vi "WS1050 16 DUT Reliability HD_Cycling Ver1.8.vi"() -> ()   [LabVIEW 2012]
uses:
  Type Defs/WSVCAP SHL I2C DUT Mask Mode Enum.ctl
  <vilib>/Utility/file.llb/Read From Spreadsheet File (DBL).vi
  SubVI/Agilent E363X Series/Agilent E363X Series.lvlib
  SubVI/keithley_2000/Keithley 2000/Keithley 2000.lvlib
  SubVI/2012_Keithley 24XX/Keithley 24XX.lvlib
panel:
  out "VISA resource name out":refnum<visa-resource-name>="GPIB0::3::INSTR"
  out "error out 2":errorcluster={"status"=TRUE, "code"=-63192, "source"="niLvFpga_Open_PXI-7813R.vi"}
  in  "Reg1_Bit Cntrl":string[](array[string])=["01", "02", "04", "08", "10", "20", "40", "80", "03", "06", "0C", "D8", "33", "66", "CC", "07", "0E", "1C", "38", "70", "E0", "0F", "1E", "3C", "78", "F0", "1F", "3E", "7C", "F8", "3F", "7E", "FC", "7F", "FE", "FD", "FB", "F7", "EF", "DF", "BF", "7F", "FC", "F9", "F3", "E7", "CF", "9F", "3F", "F8", "F1", "E3", "C7", "8F", "1F", "F0", "E1", "C3", "87", "0F", "E0", "C1", "83", "07", "C0", "81", "03", "AA", "55", "00"]
  out "date string":string="5/19/2014"
  out "PS1 Out":refnum<visa-resource-name>
  out "Ke2000 Out":refnum<visa-resource-name>="GPIB0::9::INSTR"
  in  "Tab Control":T1(tab)
  in  "No of Cmd":i64=3
  in  "Serial Number":string[][](table)=[["DUT", "SN"], ["DUT1", "1"], ["DUT2", "2"], ["DUT3", "3"], ["DUT4", "4"], ["DUT5", "5"], ["DUT6", "6"], ["DUT7", "7"], ["DUT8", "8"], ["DUT9", "9"], ["DUT10", "10"], ["DUT11", "11"], ["DUT12", "12"], ["DUT13", "13"], ["DUT14", "14"], ["DUT15", "15"], ["DUT16", "16"]]
  out "AD7747 Values":string[][](table)
  in  "SPI Clock Rate (Hz)":dbl=5000000.0 caption="Cycle Speed" format="%.1p Hz"
  in  "Lot#":string="3T9BB"
  in  "Wafer#":string="25-EB"
  in  "File Name":string="CYC_3T9BB_25_EB_65C_40V_50DC_BRD3_141107_1"
  in  "TMN DC\\CAP Data Log File Path":path=path "C:/WS1050 16 DUT Data"
  in  "Test Program":string="WS1050 16 DUT Reliability HD_Cycling Ver1.8"
  out "Current Date":string="8/28/2014"
  out "Current Time":string="0950"
  in  "Start Date":string="4/24/2014"
  in  "Start Time":string="1542"
  in  "Comment":string="CYC65C40V"
  in  "OK Button":bool
  in  "Calibration":bool
  in  "Verify CP":bool
  in  "CP Setting":i32(ring) items=["CP OFF", "CP ON", "CP 35V", "CP 40V", "DVA ON", "DVA OFF", "REG1 ON", "REG1 OFF", "REG2 ON", "REG2 OFF", "REG3 ON", "REG3 OFF"]
  in  "Set VDD":dbl=3.7 format="%.3g"
  in  "Command":string[](array[string])=["0702013B3B3B", "0702013B3B3B", "070201000000"]
  in  "SPI Clock Rate (Hz)":dbl=1000000.0 caption="Meas Speed" format="%.1p Hz"
  out "AR  Meas(Hz)":dbl
  in  "PS1 Source":refnum<visa-resource-name>="GPIB0::5::INSTR"
  in  "Ke2000":refnum<visa-resource-name>="GPIB0::9::INSTR"
  in  "CP to HD/Cycle":i32(ring)=1 items=["CP HDC 35V", "CP HDC 40.25V", "CP HDC 27.5V", "CP HDC 30.5V", "CP HDC 44V"]
  out "Simulate FPGA":bool
  out "Online":bool
  out "AR Cycling(Hz)":dbl=5000000.0
  in  "Ke2400":refnum<visa-resource-name>="GPIB0::3::INSTR"
  in  "Initialize AD7747":bool
  in  "DUT Mask Mode":T2=enum."All"
  in  "RFFE Slave Address":u8=7 caption="Slave Address" format="0x%02x"
  out "Activity Log":string="05/19/2014 -- 12:24:35.853::WSVCAP::APP::Application Started\n05/19/2014 -- 12:24:37.606::WSVCAP::WSVCAP SHL::WR I2C-REG:0x0A;MASK:0xFFFFFFFFFFFF;C1 DATA:22:22:22:22:22:22:22:22:22:22:22:22:22:22:22:22;C2 DATA:22:22:22:22:22:22:22:22:22:22:22:22:22:22:22:22;C3 DATA:22:22:22:22:22:22:22:22:22:22:22:22:22:22:22:22\r\n05/19/2014 -- 12:24:37.773::WSVCAP::WSVCAP SHL::WR I2C-ST:0,0,4,1\r\n05/19/2014 -- 12:24:37.903::WSVCAP::WSVCAP SHL::RD I2C-BYTES:4;ADD:0x00;MASK:0xFFFFFFFFFFFF\r\n05/19/2014 -- 12:24:38.045::WSVCAP::WSVCAP SHL::RD I2C:C1 DATA:2:2:2:2:2:2:2:2:2:2:2:2:2:2:2:2|A7:A9:AA:82:82:7F:82:81:82:81:83:82:81:82:82:81|46:36:BB:88:44:A3:E9:2B:32:20:ED:25:BB:3D:68:B|2C:6A:EB:A7:22:56:FE:CC:36:82:D7:B0:3B:48:F9:CC;C2 DATA:2:2:2:2:2:2:2:2:2:2:2:2:2:2:2:2|94:94:94:80:80:80:80:80:81:7E:7E:81:80:7E:80:80|47:33:15:82:62:B:E8:1C:D7:C3:7D:41:7C:B7:4C:2A|C4:B4:AE:8:1E:D1:4E:37:11:C0:6F:63:42:9D:63:B5;C3 DATA:2:2:2:2:2:2:2:2:2:2:2:2:2:2:2:2|95:95:95:81:81:7E:81:80:84:7D:80:83:81:7E:7F:80|AB:C4:14:B5:7B:52:DF:C9:79:5D:5F:30:99:31:1E:F4|6E:5C:F7:A8:C3:EB:7B:EF:33:92:89:77:4D:67:75:DD;STATUS:0:0:4:0\r\n05/19/2014 -- 12:24:38.046::WSVCAP::WSVCAP SHL::WR I2C-REG:0x0A;MASK:0xFFFFFFFFFFFF;C1 DATA:22:22:22:22:22:22:22:22:22:22:22:22:22:22:22:22;C2 DATA:22:22:22:22:22:22:22:22:22:22:22:22:22:22:22:22;C3 DATA:22:22:22:22:22:22:22:22:22:22:22:22:22:22:22:22\r\n05/19/2014 -- 12:24:38.089::WSVCAP::WSVCAP SHL::WR I2C-ST:0,0,4,1\r\n05/19/2014 -- 12:24:38.219::WSVCAP::WSVCAP SHL::RD I2C-BYTES:4;ADD:0x00;MASK:0xFFFFFFFFFFFF\r\n05/19/2014 -- 12:24:38.362::WSVCAP::WSVCAP SHL::RD I2C:C1 DATA:2:2:2:2:2:2:2:2:2:2:2:2:2:2:2:2|A7:AB:AA:82:82:82:83:83:82:82:82:82:7F:82:82:81|4B:32:96:83:3E:61:43:17:25:62:AB:4D:A2:40:2E:5|3C:76:2B:B4:EE:E4:A9:1A:AA:A:26:C7:21:2E:87:5B;C2 DATA:2:2:2:2:2:2:2:2:2:2:2:2:2:2:2:2|94:94:94:80:80:80:80:80:80:7F:80:81:80:80:7F:80|4A:32:19:7D:19:6C:79:46:61:7F:4B:B8:A5:30:F3:14|B4:70:A:8C:9C:DC:43:FA:1E:A:C6:21:A:A9:13:F3;C3 DATA:2:2:2:2:2:2:2:2:2:2:2:2:2:2:2:2|95:97:94:81:80:81:82:81:80:7E:81:84:7F:81:80:80|B2:32:D0:A7:9E:4C:AB:D4:EE:D9:F0:82:B7:91:7:FF|C1:91:B6:3D:D8:E:1B:4F:9F:6A:F1:6C:E7:3F:7:BA;STATUS:0:0:4:0\r\n05/19/2014 -- 12:24:38.364::WSVCAP::WSVCAP SHL::WR I2C-REG:0x0A;MASK:0xFFFFFFFFFFFF;C1 DATA:22:22:22:22:22:22:22:22:22:22:22:22:22:22:22:22;C2 DATA:22:22:22:22:22:22:22:22:22:22:22:22:22:22:22:22;C3 DATA:22:22:22:22:22:22:22:22:22:22:22:22:22:22:22:22\r\n05/19/2014 -- 12:24:38.406::WSVCAP::WSVCAP SHL::WR I2C-ST:0,0,4,1\r\n05/19/2014 -- 12:24:38.536::WSVCAP::WSVCAP SHL::RD I2C-BYTES:4;ADD:0x00;MASK:0xFFFFFFFFFFFF\r\n05/19/2014 -- 12:24:38.678::WSVCAP::WSVCAP SHL::RD I2C:C1 DATA:2:2:2:2:2:2:2:2:2:2:2:2:2:2:2:2|A7:A9:AB:82:82:81:82:82:82:82:82:82:82:82:82:81|46:71:4C:87:43:3D:7F:FC:25:4F:8E:54:97:3E:60:8C|AA:F4:1F:B5:CE:43:1F:36:9:87:9C:78:86:5:B6:8E;C2 DATA:2:2:2:2:2:2:2:2:2:2:2:2:2:2:2:2|94:94:94:80:7F:7F:80:80:80:80:80:81:80:80:80:80|49:36:18:7D:6E:C5:E4:3C:81:2E:41:D3:75:71:E3:72|E8:D3:E6:D1:E0:48:AE:D4:54:D:E8:8E:B4:41:68:4;C3 DATA:2:2:2:2:2:2:2:2:2:2:2:2:2:2:2:2|95:95:95:81:7F:7F:81:81:81:81:81:84:81:81:82:81|B3:F5:90:AB:82:69:7B:93:D0:77:E8:D5:E8:8C:84:E8|B9:AC:EE:2B:B6:71:8F:4A:74:31:56:BB:8A:B7:A0:C8;STATUS:0:0:4:0\r\n05/19/2014 -- 12:24:38.681::WSVCAP::WSVCAP SHL::WR I2C-REG:0x0A;MASK:0xFFFFFFFFFFFF;C1 DATA:22:22:22:22:22:22:22:22:22:22:22:22:22:22:22:22;C2 DATA:22:22:22:22:22:22:22:22:22:22:22:22:22:22:22:22;C3 DATA:22:22:22:22:22:22:22:22:22:22:22:22:22:22:22:22\r\n05/19/2014 -- 12:24:38.723::WSVCAP::WSVCAP SHL::WR I2C-ST:0,0,4,1\r\n05/19/2014 -- 12:24:38.854::WSVCAP::WSVCAP SHL::RD I2C-BYTES:4;ADD:0x00;MASK:0xFFFFFFFFFFFF\r\n05/19/2014 -- 12:24:38.996::WSVCAP::WSVCAP SHL::RD I2C:C1 DATA:2:2:2:2:2:2:2:2:2:2:2:2:2:2:2:2|A7:A9:AA:82:82:7F:83:81:82:81:84:82:7F:82:7F:82|43:FB:E:7F:3C:AD:35:35:26:A2:6C:21:4B:3D:8:6|63:9A:E1:F3:95:32:91:42:90:3C:78:1F:5C:D7:5F:D8;C2 DATA:2:2:2:2:2:2:2:2:2:2:2:2:2:2:2:2|94:94:94:80:80:80:80:80:81:80:7E:81:80:7E:7F:80|48:36:18:7F:5E:3D:69:83:DE:AE:A1:9E:31:AE:BB:96|15:A0:44:17:13:FD:CC:C8:6D:B2:EF:A7:C:C7:3B:F;C3 DATA:2:2:2:2:2:2:2:2:2:2:2:2:2:2:2:2|95:96:94:81:81:7E:82:80:84:80:80:84:7F:7E:7D:82|AD:3B:6D:A9:7C:57:9D:F5:7A:96:23:5C:36:2D:ED:5A|CD:46:DB:3B:C7:BD:70:60:33:B8:B:F7:63:A:51:4D;STATUS:0:0:4:0\r\n05/19/2014 -- 12:24:38.998::WSVCAP::WSVCAP SHL::WR I2C-REG:0x0A;MASK:0xFFFFFFFFFFFF;C1 DATA:22:22:22:22:22:22:22:22:22:22:22:22:22:22:22:22;C2 DATA:22:22:22:22:22:22:22:22:22:22:22:22:22:22:22:22;C3 DATA:22:22:22:22:22:22:22:22:22:22:22:22:22:22:22:22\r\n05/19/2014 -- 12:24:39.040::WSVCAP::WSVCAP SHL::WR I2C-ST:0,0,4,1\r\n05/19/2014 -- 12:24:39.170::WSVCAP::WSVCAP SHL::RD I2C-BYTES:4;ADD:0x00;MASK:0xFFFFFFFFFFFF\r\n05/19/2014 -- 12:24:39.311::WSVCAP::WSVCAP SHL::RD I2C:C1 DATA:2:2:2:2:2:2:2:2:2:2:2:2:2:2:2:2|A7:AA:AB:82:82:81:82:81:82:81:82:82:82:82:7F:82|44:F1:90:87:45:44:C8:2C:2C:F1:FC:1B:94:3B:3C:75|4A:49:95:19:99:73:64:3:23:24:F3:A2:5E:7F:C4:B6;C2 DATA:2:2:2:2:2:2:2:2:2:2:2:2:2:2:2:2|94:94:94:80:80:80:80:7F:80:80:7E:80:80:7E:7F:80|4C:36:17:7D:A8:9F:DE:C7:53:6D:8A:F4:41:A5:C6:E0|90:2E:24:C:D9:22:E4:76:3B:40:1D:53:33:B1:3E:4D;C3 DATA:2:2:2:2:2:2:2:2:2:2:2:2:2:2:2:2|95:97:95:81:81:7F:81:80:80:81:7F:82:81:7E:7D:82|AE:2B:A7:AB:CC:CD:A4:38:FD:17:80:F2:92:2D:45:C4|76:E5:D:B9:AD:B5:BA:8D:28:32:9E:42:B7:20:4A:D9;STATUS:0:0:4:0\r\n05/19/2014 -- 12:24:39.313::WSVCAP::WSVCAP SHL::WR I2C-REG:0x0A;MASK:0xFFFFFFFFFFFF;C1 DATA:22:22:22:22:22:22:22:22:22:22:22:22:22:22:22:22;C2 DATA:22:22:22:22:22:22:22:22:22:22:22:22:22:22:22:22;C3 DATA:22:22:22:22:22:22:22:22:22:22:22:22:22:22:22:22\r\n05/19/2014 -- 12:24:39.355::WSVCAP::WSVCAP SHL::WR I2C-ST:0,0,4,1\r\n05/19/2014 -- 12:24:39.486::WSVCAP::WSVCAP SHL::RD I2C-BYTES:4;ADD:0x00;MASK:0xFFFFFFFFFFFF\r\n05/19/2014 -- 12:24:39.628::WSVCAP::WSVCAP SHL::RD I2C:C1 DATA:2:2:2:2:2:2:2:2:2:2:2:2:2:2:2:2|A7:A9:AA:82:82:82:83:82:82:82:82:82:7F:82:7F:82|47:18:E4:87:3E:E7:6:65:25:92:37:38:A8:3E:89:85|7C:A7:7:2B:A3:7A:EC:EF:89:ED:F4:D3:D8:BC:3A:F5;C2 DATA:2:2:2:2:2:2:2:2:2:2:2:2:2:2:2:2|94:94:94:80:7F:80:80:7F:81:80:7E:80:80:80:81:80|49:37:17:80:76:25:6A:F8:DF:55:97:4D:B8:5B:2B:B1|13:E3:9A:3E:1A:2D:4F:B6:DB:E9:61:FA:8B:D6:9:CC;C3 DATA:2:2:2:2:2:2:2:2:2:2:2:2:2:2:2:2|95:95:95:81:7F:80:82:81:84:80:7F:81:80:81:7F:82|AF:93:3B:AF:5B:11:82:E4:7E:C3:2D:72:9:96:D9:A|DB:96:F2:10:5F:64:9A:C6:98:12:27:7D:10:D3:20:D9;STATUS:0:0:4:0\r\n05/19/2014 -- 12:24:40.132::WSVCAP::WSVCAP SHL::CLOSE\r\n"
  in  "C1 Cap DAC":u8=128 caption="B Data In" format="0x%02x"
  in  "C2 Cap DAC":u8=128 caption="B Data In" format="0x%02x"
  in  "C3 Cap DAC":u8=128 caption="B Data In" format="0x%02x"
  out "IDD Brd(uA)":string
  in  "CP to Meas":i32(ring)=1 items=["CP HDC 35V", "CP HDC 40.25V", "CP HDC 27.5V", "CP HDC 30.5V", "CP HDC 44V"]
  in  "Set Delay":dbl[](array[numeric])=[1.8e-05, 1.8e-05, 1.8e-05] min=0.0 max=0.5 format="%#.0p s"
  in  "CP VPI":i32(ring) items=["CP HDC 35V", "CP HDC 40.25V", "CP HDC 27.5V", "CP HDC 30.5V", "CP HDC 44V"]
  in  "Real No. From\nLookup Table":bool
  in  "Control Panel":T3={"Verify Socket"=FALSE, "HD/CYC"=FALSE, "E-CAL"=FALSE, "DVA"=FALSE, "VPI"=TRUE, "VSA"=TRUE, "HS"=TRUE}
  out "Verify Socket":bool
  out "HD/CYC":bool
  out "E-CAL":bool
  out "DVA":bool
  out "VPI":bool
  out "VSA":bool
  out "HS":bool
  in  "Repeat Meas(s)":u32=300
  in  "Freq(Hz)":string="12K"
  in  "Brd #":string="1"
  out "error out":errorcluster
  in  "error in (no error)":errorcluster
  in  "WS1050/51":bool=TRUE
  in  "Test Sequences":i32(ring) items=["C1_C2_C3", "C2_C1_C3", "C3_C2_C1"]
  in  "%Duty Cycle":string="33"
  in  "Cmin/Act":bool
  in  "Cmd to HD":string="070201383838"
  out "40V_1":string[][](table)
  out "VPI C1":string[][](table)
  out "VPI C3":string[][](table)
  out "NOM IDD OFF(uA)":string
  out "40V_2":string[][](table)
  out "VPI C2":string[][](table)
  out "NOM IDD ON (uA)":string
  out "40V_3":string[][](table)
  out "Total Time":u64
  out "IDD Stdby(uA)":string="2.606990E+0"
  out "EFuse RB T0":string[](array[string])
  out "Current EFuse Read back":string[](array[string])
  in  "Set HD/Cycle \nto Complete":u64=50000000000
  out "No of HD/Cycle\nCompleted":u64
  out "Cycle Count":u64 min=1 max=4 step=1
  out "Loop \ncompleted":i32=1
  out "Previous Time":string="12:20:26 PM"
  out "STATUS":string="Idle...."
  out "IDD_HD/CYC (uA)":string="164.601255E+0"
  in  "stop During HD/Cycles":bool
  in  "stop":bool
  out "Total Delta 2(pF)":string[](array[string])
  out "Total Delta 1(pF)":string[](array[string])
  out "Total Delta 3(pF)":string[](array[string])
  out "% Delta C_T0":string[][](array[string])
  out "% Delta C":string[][](array[string])
  out "EFuse Readback Status":bool[](array[boolean])
  in  "DeltaC Target(pF)_50":dbl=7.375
  out "RB Reg for HD":string[](array[string])
  out "RB Reg for HD/Cycle":string[](array[string])
  in  "DeltaC Target(pF)_51":dbl=5.875
  out "VSA_V1":string[][](table)
  out "VSA_V2":string[][](table)
  out "VSA_V3":string[][](table)
  in  "VSA Voltage(V)":dbl[](array[numeric])=[-10.0, 0.0, 10.0]
  in  "DC_Temp":i32=65
  in  "HD/CYC Temp":i32=65
  in  "Time All ON (s)":u32=120
  in  "Time All OFF (s)":u32=120
  in  "HD_DC (Min)":u64=259200
  out "LPs Count":i32
  in  "X Repeat":i32=100
  out "No LPs to RP":i32
  out "Running Loops":i32=1
  out "TTime Completed":u64=2000
  in  "TTF Completed":u64=50000000000
  in  "HD RP(Min)":dbl=60.0
  in  "CYC RP (X1000)":dbl=10000.0
  out "Min Plot_1":dbl[][](graph) caption="(Y) Multi Plot 2"
  out "Min Plot_2":dbl[][](graph) caption="(Y) Multi Plot 2"
  out "Min Plot_3":dbl[][](graph) caption="(Y) Multi Plot 2"
  in  "Debug":bool
  in  "No of Rows\nFrom Spread Sheet":i32
  in  "Plot Delta Cmin":bool=TRUE
  in  "Plot":T4(ring)
  # "Company:  WiSpry Inc\n20 Fairbanks Ste 198 Irvine CA 92618\n\nAuthor:  Andy V Tran\nCreated:  09/14/2015\nLabVIEW 2012 Pro\nTP:  WS1050 16 DUT HD/Cycle ver1.8\nFPGA Version: WS_VCAP Driver 024"
  # "Note for HD during Cycles Setup:\n\n1.  Set HD/Cycle to Completed = 4320 minutes = 72 hours \n(T0 24hrs HD, T2 48hrs HD_Duty Cycle);  Default Setting\n2.  Set Time to Start HD Duty Cycle = 1440 = 24 hours\n3.  Set Time All ON = 120s = 2 minutes\n4.  Set Time All OFF = 120s = 2 minutes\n5.  No of Loops to RP = 3600s/(Time ALL ON(s) + Time ALL + OFF(s))\n6.  X Repeat = X runs\n7.  Set TTF Completed = Repeat X item1 to Stop.\n8.  Stop Test, set TTF Completed = Total Time Completed.\n\nNote for Cycling:\n\n\n\nVersion 1.8 is the latest verision for WS1050 16 DUT test program.\n\n1.  Added Stress Sequences,\n2.  Added CMin/ON-OFF Repeat Measurement\n3.  Fill \"na\" when no test"
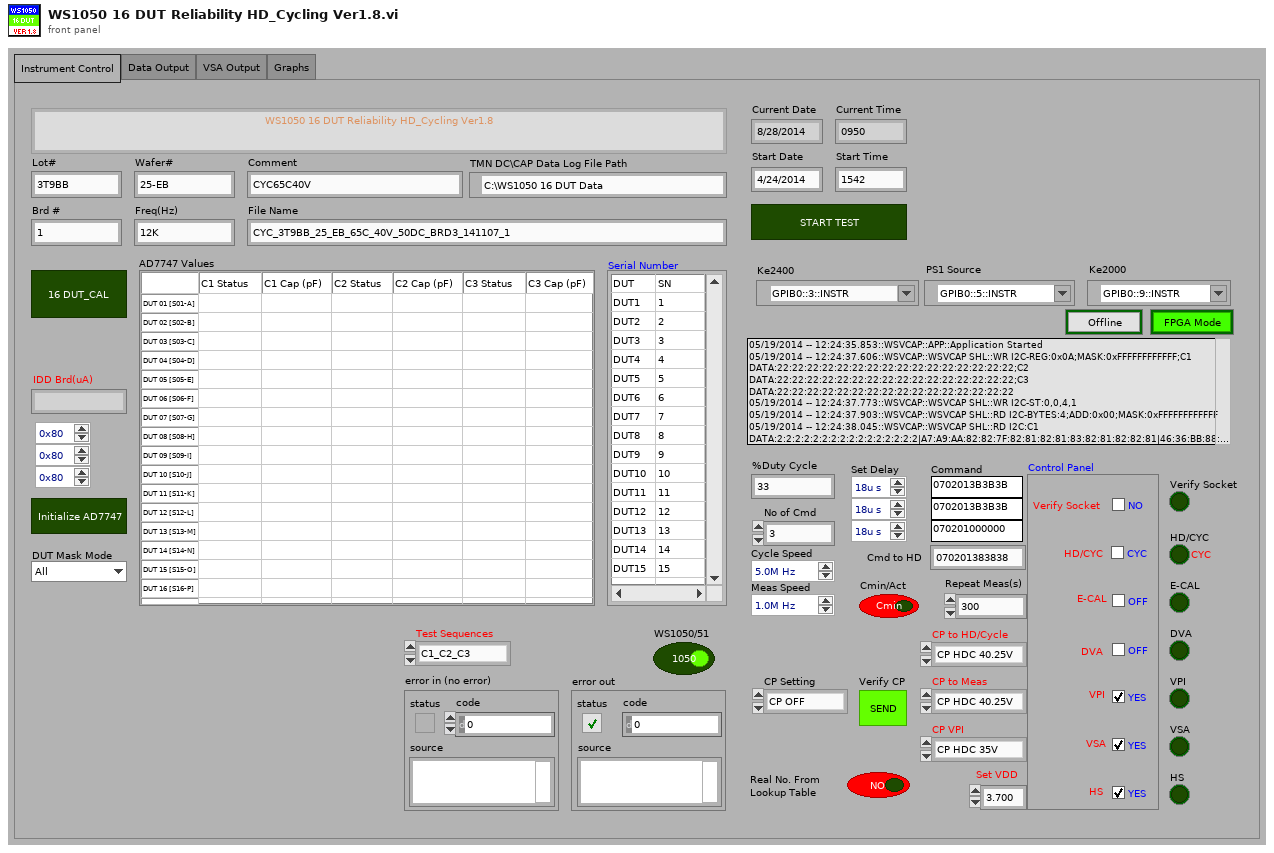
[diagram p1: front panel]
types:
  T1 = enum32{"Instrument Control", "Data Output", "VSA Output", "Graphs"}
  T2 = typedef "WSVCAP SHL I2C DUT Mask Mode Enum.ctl" = enum16{"Custom", "C1", "C2", "C3", "All"}
  T3 = cluster{"Verify Socket":bool, "HD/CYC":bool, "E-CAL":bool, "DVA":bool, "VPI":bool, "VSA":bool, "HS":bool}
  T4 = enum16{"DUT ALL", "DUT 01", "DUT 02", "DUT 03", "DUT 04", "DUT 05", "DUT 06", "DUT 07", "DUT 08", "DUT 09", "DUT 10", "DUT 11", "DUT 12", "DUT 13", "DUT 14", "DUT 15", "DUT 16"}
  T5 = typedef "WSVCAP SHL Core System Cluster.ctl" = cluster{"Settings":T6, "FPGA Resource":tag, "Online":bool, "I2C Wait Ticks":u32, "SPI Wait Ticks":u32, "RFFE Wait Ticks":u32}
  T6 = typedef "WSVCAP SHL I2C Settings Cluster.ctl" = cluster{"FPGA Resource Name":string, "I2C Slave Address":u8, "I2C Clock Rate (Hz)":dbl, "SPI Clock Rate (Hz)":dbl, "RFFE Slave Address":u8, "RFFE Clock Rate (Hz)":dbl, "Simulate FPGA":bool, "C1 Cap DAC Default":u8, "C2 Cap DAC Default":u8, "C3 Cap DAC Default":u8}
  T7 = enum16{"Idle...", "Voltage 1", "Voltage 2", "Voltage 3"}[]
  T8 = cluster{"Test Program ":string, "Comment":string, "Data Out":string, "Data Out":string, "Data Out":string, string, "Data Out":string, "Data Out":string, "string":string, "Freq(Hz)":string, "Brd #":string}
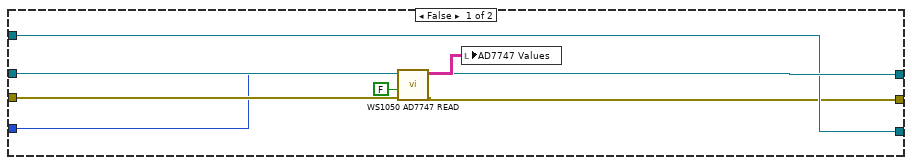
[diagram p9: hidden frame]
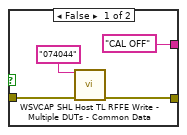
[diagram p10: hidden frame]
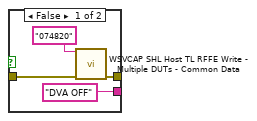
[diagram p11: hidden frame]
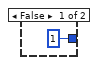
[diagram p12: hidden frame]
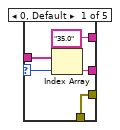
[diagram p13: hidden frame]
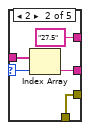
[diagram p14: hidden frame]
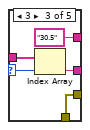
[diagram p15: hidden frame]
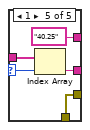
[diagram p16: hidden frame]
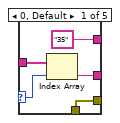
[diagram p17: hidden frame]
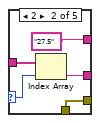
[diagram p18: hidden frame]
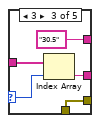
[diagram p19: hidden frame]
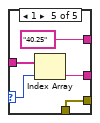
[diagram p20: hidden frame]
diagram:
  w18 = TRUE
  w24 = u16 0 items=["Off", "Moving Filter", "Repeating Filter"] ("Digital Filter (0: Off)")
  w25 = u16 7 items=["3.5 Digits"=4, "4.5 Digits"=5, "5.5 Digits"=6, "6.5 Digits"=7] ("Resolution (7: 6.5 digits)")
  n1 = case shown="True" w18 {
    tunnel: "error in (no error)" -> [w34 w35]
    tunnel: [w34 w42] -> w4
    frame False {
    }
    frame True {
      n2 = call "WSVCAP SHL Host TL Initialize.vi"("error in"=w35) -> ("error out"=w36:errorcluster)  [unwired: 13 in, 1 out]
      n3 = control-ref of="Activity Log"() -> (w38:refnum<vi>)
      n4 = call "ACT LG Activity Log Core.vi"("Display Ref"=w38, "Source"="WSVCAP", "Error In (no error)"=w36) -> ("Error Out"=w37:errorcluster)  [unwired: 11 in, 1 out]
      n5 = call "WSVCAP SHL Host TL Status Manager.vi"("error in"=w37) -> ("System Out"=w43:T5, "error out"=w42:errorcluster)  [unwired: 13 in]
      n6 = Unbundle By Name(w43) -> ("Online"=→"Online":bool, "Settings.Simulate FPGA"=→"Simulate FPGA":bool)
    }
  }
  n7 = case shown="True" TRUE {
    tunnel: w4 -> [w44 w49]
    tunnel: [w45 w48] -> w15
    tunnel: [w44 w47] -> w8
    tunnel: "Ke2400" -> [w45 w46]
    frame False {
    }
    frame True {
      n8 = VISA Write(VISA resource name=w46, write buffer="SOUR:FUNC VOLT;VOLT:MODE FIX;RANG 100;LEV 0.0;:SENS:FUNC \"CURR\";CURR:PROT 60E-3;RANG 100E-3;:OUTP ON", error in (no error)=w49) -> (VISA resource name out=w48:refnum<visa-resource-name>, error out=w47:errorcluster)  [unwired: 1 out]
    }
  }
  n9 = call "Initialize.vi"("VISA resource name"="Ke2000", "error in (no error)"=w4) -> ("VISA resource name out"=w27:refnum<visa-resource-name>, "error out"=w26:errorcluster)  [unwired: 16 in]
  n10 = call "Initialize.vi"("error in (no error)"=w4, "Reset? (T: Yes)"=FALSE, "ID Query? (T: Yes)"=TRUE, "VISA resource name"="PS1 Source") -> ("error out"=w3:errorcluster, "VISA resource name out"=w30:refnum<visa-resource-name>)  [unwired: 6 in]
  n11 = call "Configure DC Current.vi"("VISA resource name"=w27, "Resolution (7: 6.5 digits)"=w25, "error in (no error)"=w26, "Auto Range? (T: Auto)"=FALSE, "Digital Filter (0: Off)"=w24, "Custom Range (0 A)"=1.0) -> ("VISA resource name out"=w22:refnum<visa-resource-name>, "error out"=w5:errorcluster)  [unwired: 12 in]
  n12 = case shown="True" TRUE {
    tunnel: [_ w51] -> w33
    frame False {
    }
    frame True {
      n13 = call-poly <vilib>:"Read From Spreadsheet File.vi"("number of rows (all:-1)"=-1) -> ("all rows"=w51:dbl[][])  [unwired: 6 in, 4 out]
    }
  }
  n14 = Merge Errors(w8, w5, w3) -> (w16:errorcluster)
  n15 = while {
    tunnel: w16 -> [w76]
    tunnel: [w64] -> w12
    tunnel: w33 -> [w81]
    tunnel: w30 -> [w68]
    tunnel: w22 -> [w69]
    tunnel: [w79] -> w21
    tunnel: [w78] -> w20
    tunnel: w15 -> [w75]
    tunnel: [w74] -> w13
    tunnel: [FALSE ("stop")] -> w6
    i -> [w77]
    stop <- w82 stop-if-true
    n16 = case shown="0" w77 {
      tunnel: w76 -> [w92 w94]
      tunnel: [w91 w94] -> w71
      tunnel: "RFFE Slave Address" -> [w89 _]
      frame 0 {
        w85 = dbl[][] []
        w84 = "" ("uA")
        w86 = string[][] []
        w87 = string[] [] ("EFuse Read back")
        w93 = u64 0 ("No of HD/Cycle\nCompleted")
        n17 = local write "RB Reg for HD/Cycle"(w87) -> ()
        n18 = local write "Current EFuse Read back"(w87) -> ()
        n19 = local write "EFuse RB T0"(w87) -> ()
        n20 = local write "No of HD/Cycle\nCompleted"(w93) -> ()
        n21 = local write "Cycle Count"(w93) -> ()
        n22 = local write "Total Delta 1(pF)"(w87) -> ()
        n23 = local write "Total Delta 2(pF)"(w87) -> ()
        n24 = local write "Total Delta 3(pF)"(w87) -> ()
        n25 = local write "VPI C2"(w86) -> ()
        n26 = local write "VSA_V3"(w86) -> ()
        n27 = local write "VSA_V1"(w86) -> ()
        n28 = local write "VSA_V2"(w86) -> ()
        n29 = local write "VPI C1"(w86) -> ()
        n30 = local write "VPI C3"(w86) -> ()
        n31 = local write "% Delta C"(w86) -> ()
        n32 = local write "% Delta C_T0"(w86) -> ()
        n33 = local write "40V_2"(w86) -> ()
        n34 = local write "40V_1"(w86) -> ()
        n35 = local write "40V_3"(w86) -> ()
        n36 = local write "NOM IDD OFF(uA)"(w84) -> ()
        n37 = local write "NOM IDD ON (uA)"(w84) -> ()
        n38 = local write "IDD Brd(uA)"(w84) -> ()
        n39 = local write "Min Plot_3"(w85) -> ()
        n40 = local write "Min Plot_1"(w85) -> ()
        n41 = local write "Min Plot_2"(w85) -> ()
        n42 = call "WSVCAP SHL Host TL RFFE Configure.vi"("RFFE Slave Address"=w89, "Clock Rate (Hz)"="SPI Clock Rate (Hz)", "error in"=w92) -> ("Actual Rate (Hz)"=→"AR  Meas(Hz)":dbl, "error out"=w91:errorcluster)  [unwired: 11 in]
      }
      frame 1, Default {
      }
    }
    n43 = while {
      tunnel: ["stop"] -> w73
      tunnel: w71 -> [w119]
      tunnel: [w110] -> w65
      tunnel: w68 -> [w117]
      tunnel: w69 -> [w112]
      tunnel: [w113] -> w67
      tunnel: [w111] -> w66
      tunnel: [w106] -> w63
      tunnel: [w105] -> w62
      tunnel: [w104] -> w61
      tunnel: [w103] -> w60
      tunnel: [w102] -> w59
      tunnel: [w101] -> w58
      tunnel: [w100] -> w57
      tunnel: ["Command"] -> w56
      tunnel: ["Set Delay"] -> w55
      stop <- w126 stop-if-true
      # "Set Date & Time to Start Test"
      n44 = case shown="True" "Initialize AD7747" {
        tunnel: w119 -> [w135 w140]
        tunnel: [w135 w136] -> w118
        tunnel: w117 -> [w134 w138]
        tunnel: [w134 w137] -> w116
        frame False {
        }
        frame True {
          w141 = T7 [enum."Voltage 2", enum."Voltage 3", enum."Voltage 1"] items=["Idle...", "Voltage 1", "Voltage 2", "Voltage 3"]
          n45 = for {
            tunnel: w138 -> [w151]
            tunnel: w141 -> [w148] mode=indexing
            tunnel: [w147] -> w137
            shift-right: [w143] -> w139
            shift-left: w140 -> [w152]
            n46 = local read "Set VDD"() -> (w146:dbl)
            n47 = call "E3631A_Voltage Controller.vi"("VISA resource name"=w151, "I_VDD(A)"=0.2, "Channel Controller"=w148, "Voltage 1"=w146, "Voltage 2"=3.3, "error in (no error)"=w152, "Voltage 3"=-3.3) -> ("VISA resource name out"=w147:refnum<visa-resource-name>, "error out"=w142:errorcluster)  [unwired: 7 in]
            n48 = call "Delay T4.vi"("milliseconds to wait"=u32 100, "error in (no error)"=w142) -> ("error out"=w143:errorcluster)  [unwired: 9 in]
          }
          n49 = call "WS1050_AD7747_Init.vi"("error in"=w139) -> ("error out"=w136:errorcluster)  [unwired: 10 in]
        }
      }
      n50 = call "Time_stamp.vi"() -> ("date/time string"=w131:string, "date string"=w133:string)  [unwired: 2 in]
      "Current Date" <- w133
      "Current Time" <- w131
      n51 = Equal?(x=w133, y="Start Date") -> (x = y?=w129:bool)
      n52 = Equal?(x=w131, y="Start Time") -> (x = y?=w128:bool)
      n53 = And(x=w129, y=w128) -> (x .and. y?=w125:bool)
      n54 = Compound Arithmetic op=OR(w125, "OK Button", "stop") -> (w126:bool)
      n55 = case shown="True" "Calibration" {
        tunnel: w118 -> [w181 w199]
        tunnel: [w176 w196] -> w108
        tunnel: w116 -> [w180 w195]
        tunnel: "DUT Mask Mode" -> [w179 w191]
        tunnel: [w180 w190] -> w114
        tunnel: w112 -> [w178 w186]
        tunnel: [w178 w183] -> w111
        frame False {
          n56 = call "WS1050 AD7747 READ.vi"("error in"=w181, "Log (T)"=FALSE, "DUT Mask Mode (All)"=w179) -> ("error out"=w176:errorcluster, "AD7747 Values"=w182:string[][])  [unwired: 7 in]
          n57 = local write "AD7747 Values"(w182) -> ()
        }
        frame True {
          n58 = flat-sequence {
            tunnel: w199 -> [w208]
            tunnel: [w203] -> w198
            tunnel: w195 -> [w207]
            tunnel: [w206] -> w194
            tunnel: w191 -> [w205]
            tunnel: [w205] -> w192
            tunnel: w186 -> [w201]
            tunnel: [w200] -> w185
            tunnel: w198 -> [w236]
            tunnel: [w223] -> w197
            tunnel: w194 -> [w235]
            tunnel: [w235] -> w193
            tunnel: w192 -> [w234]
            tunnel: "C1 Cap DAC" -> [w230]
            tunnel: "C2 Cap DAC" -> [w229]
            tunnel: "C3 Cap DAC" -> [w228]
            tunnel: w185 -> [w227]
            tunnel: [w227] -> w184
            tunnel: w197 -> [w239]
            tunnel: [w242] -> w196
            tunnel: w193 -> [w241]
            tunnel: [w238] -> w190
            tunnel: w184 -> [w237]
            tunnel: [w237] -> w183
            frame #0 {
              w209 = T7 [enum."Voltage 2", enum."Voltage 3", enum."Voltage 1"] items=["Idle...", "Voltage 1", "Voltage 2", "Voltage 3"]
              n59 = for {
                tunnel: w207 -> [w220]
                tunnel: w209 -> [w217] mode=indexing
                tunnel: [w216] -> w206
                shift-right: [w214] -> w202
                shift-left: w208 -> [w221]
                n60 = local read "Set VDD"() -> (w211:dbl)
                n61 = call "E3631A_Voltage Controller.vi"("VISA resource name"=w220, "I_VDD(A)"=0.2, "Channel Controller"=w217, "Voltage 1"=w211, "Voltage 2"=3.3, "error in (no error)"=w221, "Voltage 3"=-3.3) -> ("VISA resource name out"=w216:refnum<visa-resource-name>, "error out"=w213:errorcluster)  [unwired: 7 in]
                n62 = call "Delay T4.vi"("milliseconds to wait"=u32 100, "error in (no error)"=w213) -> ("error out"=w214:errorcluster)  [unwired: 9 in]
              }
              n63 = call "Ke2000 Reading MilAmp.vi"("error in (no error)"=w202, "VISA resource name"=w201) -> ("error out"=w203:errorcluster, "uA"=→"IDD Brd(uA)":string, "VISA resource name out"=w200:refnum<visa-resource-name>)  [unwired: 7 in]
              n64 = One Button Dialog(message="Please verify all sockets should be empty...") -> ()  [unwired: 1 in, 1 out]
            }
            frame #1 {
              # "Calibration Multi-Sockets"
              n65 = call "WS1050 CAPDAC Setting.vi"("DUT Mask Mode (All)"=w234, "error in"=w236, "C3 Cap DAC"=w228, "C2 Cap DAC"=w229, "C1 Cap DAC"=w230) -> ("error out"=w232:errorcluster)  [unwired: 5 in, 1 out]
              n66 = call "WS1050 OFFSET CAL.vi"("error in"=w232, "OFFSET CAL"=TRUE ("Read?")) -> ("error out"=w231:errorcluster)  [unwired: 8 in, 1 out]
              n67 = call "WS1050 AD7747 READ.vi"("error in"=w231, "Log (T)"=FALSE, "DUT Mask Mode (All)"=w234) -> ("error out"=w224:errorcluster, "AD7747 Values"=→"AD7747 Values":string[][])  [unwired: 7 in]
              n68 = call "Delay T4.vi"("milliseconds to wait"=u32 50, "error in (no error)"=w224) -> ("error out"=w223:errorcluster)  [unwired: 9 in]
            }
            frame #2 {
              w240 = T7 [enum."Voltage 2", enum."Voltage 3", enum."Voltage 1"] items=["Idle...", "Voltage 1", "Voltage 2", "Voltage 3"]
              n69 = for {
                tunnel: w241 -> [w254]
                tunnel: w240 -> [w250] mode=indexing
                tunnel: [w249] -> w238
                shift-right: [w245] -> w242
                shift-left: w239 -> [w251]
                n70 = call "E3631A_Voltage Controller.vi"("VISA resource name"=w254, "I_VDD(A)"=0.2, "Channel Controller"=w250, "Voltage 1"=0.0, "Voltage 2"=3.3, "error in (no error)"=w251, "Voltage 3"=-3.3) -> ("VISA resource name out"=w249:refnum<visa-resource-name>, "error out"=w244:errorcluster)  [unwired: 7 in]
                n71 = call "Delay T4.vi"("milliseconds to wait"=u32 100, "error in (no error)"=w244) -> ("error out"=w245:errorcluster)  [unwired: 9 in]
              }
              n72 = One Button Dialog(message="Calibration Completed....") -> ()  [unwired: 1 in, 1 out]
            }
          }
        }
      }
      n73 = call "Control Panel.vi"("error in (no error)"=w108, "Control Panel"="Control Panel") -> ("error out"=w107:errorcluster, "VPI"=w102:bool, "DVA"=w103:bool, "E-CAL"=w104:bool, "VSA"=w101:bool, "HD/CYC"=w105:bool, "HS"=w100:bool, "Verify Socket"=w106:bool)  [unwired: 2 in]
      "Verify Socket" <- w106
      "HS" <- w100
      "VSA" <- w101
      "VPI" <- w102
      "E-CAL" <- w104
      "HD/CYC" <- w105
      "DVA" <- w103
      n74 = case shown="True" "Verify CP" {
        tunnel: [w153 w156] -> w110
        tunnel: w114 -> [w154 w161]
        tunnel: [w154 w159] -> w113
        tunnel: w107 -> [w153 w158]
        frame False {
        }
        frame True {
          w162 = T7 [enum."Voltage 2", enum."Voltage 3", enum."Voltage 1"] items=["Idle...", "Voltage 1", "Voltage 2", "Voltage 3"]
          # "Verify CP"
          n75 = for {
            tunnel: w161 -> [w174]
            tunnel: w162 -> [w171] mode=indexing
            shift-right: [w168] -> w160
            shift-left: w158 -> [w175]
            tunnel: [w166] -> w159
            n76 = local read "Set VDD"() -> (w170:dbl)
            n77 = call "E3631A_Voltage Controller.vi"("VISA resource name"=w174, "Channel Controller"=w171, "Voltage 1"=w170, "Voltage 2"=3.3, "error in (no error)"=w175, "Voltage 3"=-3.3) -> ("VISA resource name out"=w166:refnum<visa-resource-name>, "error out"=w169:errorcluster)  [unwired: 8 in]
            n78 = call "Delay T4.vi"("milliseconds to wait"=u32 100, "error in (no error)"=w169) -> ("error out"=w168:errorcluster)  [unwired: 9 in]
          }
          n79 = Index Array(array=string[] ["074000", "074040", "07476F", "074776", "074800", "074820", "07413B", "074100", "07423B", "074200", "07433B", "074300"], index="CP Setting") -> (element=w163:string)
          n80 = call "WSVCAP SHL Host TL RFFE Write - Multiple DUTs - Common Data.vi"("Data Out"=w163, "error in"=w160) -> ("error out"=w157:errorcluster)  [unwired: 13 in]
          n81 = call "Delay T4.vi"("milliseconds to wait"=u32 10, "error in (no error)"=w157) -> ("error out"=w156:errorcluster)  [unwired: 9 in]
        }
      }
      n82 = Array Subset(array="Set Delay", length="No of Cmd") -> (w97:dbl[])  [unwired: 1 in]
      n83 = Array Subset(array="Command", length="No of Cmd") -> (w98:string[])  [unwired: 1 in]
      n84 = property on="Command" class="Arr (strict)"("Number of Rows"="No of Cmd") -> ()  [unwired: 2 in, 2 out]
      n85 = property on="Set Delay" class="Arr (strict)"("Number of Rows"="No of Cmd") -> ()  [unwired: 2 in, 2 out]
      n86 = local write "Command"(w98) -> ()
      n87 = local write "Set Delay"(w97) -> ()
      n88 = Wait Until Next ms Multiple(millisecond multiple=u32 100) -> ()  [unwired: 1 out]
    }
    n89 = case shown="False" w73 {
      tunnel: w65 -> [w312 w1843]
      tunnel: [w296 w1843] -> w64
      tunnel: w81 -> [w313 _]
      tunnel: w67 -> [w311 w1841]
      tunnel: w66 -> [w302 w1842]
      tunnel: [w309 w1842] -> w79
      tunnel: [w306 w1841] -> w78
      tunnel: w75 -> [w299 w1840]
      tunnel: [w295 w1840] -> w74
      tunnel: "RFFE Slave Address" -> [w290 _]
      tunnel: [w255 FALSE ("stop During HD/Cycles")] -> w53
      tunnel: w63 -> [w264 _]
      tunnel: w62 -> [w263 _]
      tunnel: w61 -> [w262 _]
      tunnel: w60 -> [w261 _]
      tunnel: w59 -> [w260 _]
      tunnel: w58 -> [w259 _]
      tunnel: w57 -> [w258 _]
      tunnel: w56 -> [w257 _]
      tunnel: w55 -> [w256 _]
      frame False {
        w291 = u64 0 ("Total Completed")
        w270 = u32 100 ("milliseconds to wait")
        w308 = T7 [enum."Voltage 2", enum."Voltage 3", enum."Voltage 1"] items=["Idle...", "Voltage 1", "Voltage 2", "Voltage 3"]
        w310 = T7 [enum."Voltage 2", enum."Voltage 3", enum."Voltage 1"] items=["Idle...", "Voltage 1", "Voltage 2", "Voltage 3"]
        # "DVA"
        # "Verify Socket"
        # "E-CAL"
        # "VSA"
        # "VPI"
        # "HS"
        # "DVA"
        # "HD/CYC"
        n90 = for {
          tunnel: w312 -> [w1838]
          tunnel: w311 -> [w1837]
          tunnel: w310 -> [w1834] mode=indexing
          tunnel: [w1829] -> w304
          tunnel: [w1833] -> w294
          n91 = local read "Set VDD"() -> (w1832:dbl)
          n92 = call "E3631A_Voltage Controller.vi"("VISA resource name"=w1837, "I_VDD(A)"=0.2, "Channel Controller"=w1834, "Voltage 1"=w1832, "Voltage 2"=3.3, "error in (no error)"=w1838, "Voltage 3"=-3.3) -> ("VISA resource name out"=w1833:refnum<visa-resource-name>, "error out"=w1830:errorcluster)  [unwired: 7 in]
          n93 = call "Delay T4.vi"("milliseconds to wait"=u32 100, "error in (no error)"=w1830) -> ("error out"=w1829:errorcluster)  [unwired: 9 in]
        }
        n94 = local write "TTime Completed"(w291) -> ()
        n95 = local write "Total Time"(w291) -> ()
        n96 = call "WSVCAP SHL Host TL RFFE Write - Multiple DUTs - Common Data.vi"("Data Out"="074000", "error in"=w304) -> ("error out"=w305:errorcluster)  [unwired: 13 in]
        n97 = local read "IDD Brd(uA)"() -> (w278:string)
        n98 = call "Delay T4.vi"("milliseconds to wait"=w270, "error in (no error)"=w305) -> ("error out"=w303:errorcluster)  [unwired: 9 in]
        n99 = Number To Fractional String(number="Set VDD", precision (6)=i16 2) -> (F-format string=w284:string)  [unwired: 2 in]
        n100 = call "Ke2000 Reading MilAmp.vi"("error in (no error)"=w303, "VISA resource name"=w302) -> ("error out"=w280:errorcluster, "uA"=w282:string, "VISA resource name out"=w301:refnum<visa-resource-name>)  [unwired: 7 in]
        n101 = call "Substration.vi"("error in (no error)"=w280, "Input2"=w278, "Input1"=w282) -> ("error out"=w279:errorcluster, "In1 - In2"=w281:string)  [unwired: 7 in]
        "IDD Stdby(uA)" <- w281
        n102 = call "WSVCAP SHL Host TL RFFE Write - Multiple DUTs - Common Data.vi"("Data Out"="074040", "error in"=w279) -> ("error out"=w265:errorcluster)  [unwired: 13 in]
        n103 = call "Delay T4.vi"("milliseconds to wait"=w270, "error in (no error)"=w265) -> ("error out"=w288:errorcluster)  [unwired: 9 in]
        n104 = case shown="True" w261 {
          tunnel: w288 -> [w335 w336]
          tunnel: [w334 w337] -> w286
          tunnel: ["DVA OFF" ("Data Out") "DVA ON" ("Data Out")] -> w287
          frame False {
            n105 = call "WSVCAP SHL Host TL RFFE Write - Multiple DUTs - Common Data.vi"("Data Out"="074820", "error in"=w335) -> ("error out"=w334:errorcluster)  [unwired: 13 in]
          }
          frame True {
            n106 = call "WSVCAP SHL Host TL RFFE Write - Multiple DUTs - Common Data.vi"("Data Out"="074800", "error in"=w336) -> ("error out"=w337:errorcluster)  [unwired: 13 in]
          }
        }
        n107 = for {
          N: 16 -> [_]
          tunnel: "Serial Number" -> [w318]
          tunnel: [w316] -> w267 mode=indexing
          i -> [w315]
          n108 = Increment(x=w315) -> (x+1=w314:i32)
          n109 = Index Array(array=w318, index (row)=w314, index (col)=1 ("disabled index (col)")) -> (element=w316:string)
        }
        n110 = case shown="True" w263 {
          tunnel: [1 ("X Repeat") w341] -> w293
          frame False {
          }
          frame True {
            n111 = local read "X Repeat"() -> (w341:i32)
          }
        }
        n112 = Not(x=w258) -> (.not. x?=w266:bool)
        n113 = call "Delay T4.vi"("milliseconds to wait"=w270, "error in (no error)"=w286) -> ("error out"=w273:errorcluster)  [unwired: 9 in]
        n114 = case shown="True" w262 {
          tunnel: w273 -> [w322 w324]
          tunnel: [w319 w323] -> w272
          tunnel: ["CAL OFF" ("Data Out") "CAL ON" ("Data Out")] -> w274
          frame False {
            n115 = call "WSVCAP SHL Host TL RFFE Write - Multiple DUTs - Common Data.vi"("Data Out"="074044", "error in"=w322) -> ("error out"=w319:errorcluster)  [unwired: 13 in]
          }
          frame True {
            n116 = for {
              tunnel: string[] ["074920", "074900"] -> [w331] mode=indexing
              tunnel: w324 -> [w328]
              tunnel: [w327] -> w323
              n117 = call "WSVCAP SHL Host TL RFFE Write - Multiple DUTs - Common Data.vi"("Data Out"=w331, "error in"=w328) -> ("error out"=w330:errorcluster)  [unwired: 13 in]
              n118 = call "Delay T4.vi"("milliseconds to wait"=u32 10, "error in (no error)"=w330) -> ("error out"=w327:errorcluster)  [unwired: 9 in]
            }
          }
        }
        n119 = for {
          N: w293 -> [_]
          tunnel: w313 -> [w380]
          tunnel: [w376] -> w309
          tunnel: [w375] -> w307
          tunnel: w281 -> [w374]
          tunnel: w301 -> [w373]
          tunnel: "TMN DC\\CAP Data Log File Path" -> [w372]
          tunnel: w299 -> [w370]
          tunnel: [w369] -> w297
          tunnel: w294 -> [w368]
          shift-right: [w363] -> _
          shift-left: u64 0 -> [w365]
          tunnel: w263 -> [w362]
          tunnel: w290 -> [w358]
          tunnel: w290 -> [w357]
          tunnel: w287 -> [w356]
          tunnel: w284 -> [w355]
          tunnel: [w354] -> w277
          tunnel: w274 -> [w353]
          tunnel: w272 -> [w352]
          tunnel: w261 -> [w351]
          tunnel: w264 -> [w349]
          tunnel: w260 -> [w348]
          tunnel: w266 -> [w347]
          tunnel: w259 -> [w346]
          tunnel: w267 -> [w345]
          tunnel: w257 -> [w344]
          tunnel: w256 -> [w343]
          tunnel: [w342] -> w255
          i -> [w361]
          stop <- w350 stop-if-true
          n120 = while {
            tunnel: w380 -> [w606]
            tunnel: w372 -> [w617]
            tunnel: "Lot#" -> [w616]
            tunnel: "Wafer#" -> [w615]
            tunnel: w345 -> [w614]
            tunnel: "Test Program" -> [w613]
            tunnel: w345 -> [w612]
            tunnel: "Comment" -> [w611]
            tunnel: "Lot#" -> [w610]
            tunnel: "Wafer#" -> [w609]
            tunnel: w373 -> [w605]
            tunnel: [w608] -> w376
            tunnel: [w598] -> w375
            tunnel: w374 -> [w604]
            tunnel: w370 -> [w601]
            tunnel: [w600] -> w369
            tunnel: w368 -> [w599]
            tunnel: [w505] -> w342
            tunnel: w361 -> [w543]
            tunnel: [w534] -> w363
            tunnel: w365 -> [w533]
            shift-right: [w532] -> _
            shift-left: u64 0 -> [w426]
            tunnel: [w531] -> w359
            tunnel: w362 -> [w529]
            tunnel: w358 -> [w504]
            tunnel: w357 -> [w502]
            tunnel: w356 -> [w450]
            tunnel: w355 -> [w448]
            tunnel: [w423] -> w354
            tunnel: w353 -> [w430]
            tunnel: w352 -> [w429]
            tunnel: w351 -> [w428]
            tunnel: w349 -> [w420]
            tunnel: w348 -> [w419]
            tunnel: w347 -> [w414]
            tunnel: w346 -> [w408]
            tunnel: w344 -> [w382]
            tunnel: w343 -> [w381]
            i -> [w530]
            stop <- w544 stop-if-true
            n121 = case shown="4" "CP to HD/Cycle" {
              selector: "CP to HD/Cycle" -> [w621 w626 w631 w636 w640]
              tunnel: string[] ["07476F", "074776", "074765", "074769", "07477B"] -> [w622 w627 w632 w637 w642]
              tunnel: [w620 w625 w630 w635 w641] -> w445
              tunnel: ["35.0" ("Data Out") "27.5" ("Data Out") "30.5" ("Data Out") "44.0" ("Data Out") "40.25" ("Data Out")] -> w444
              tunnel: [w618 w623 w628 w633 w638] -> w443
              tunnel: w429 -> [w618 w623 w628 w633 w638]
              frame 0, Default {
                n122 = Index Array(array=w622, index=w621) -> (element=w620:string)
              }
              frame 2 {
                n123 = Index Array(array=w627, index=w626) -> (element=w625:string)
              }
              frame 3 {
                n124 = Index Array(array=w632, index=w631) -> (element=w630:string)
              }
              frame 4 {
                n125 = Index Array(array=w637, index=w636) -> (element=w635:string)
              }
              frame 1 {
                n126 = Index Array(array=w642, index=w640) -> (element=w641:string)
              }
            }
            n127 = flat-sequence {
              tunnel: [w710] -> w597
              tunnel: [w655] -> w596
              tunnel: w606 -> [w708]
              tunnel: [w707] -> w595
              tunnel: w605 -> [w684]
              tunnel: w604 -> [w706]
              tunnel: [w706] -> w594
              tunnel: [w649] -> w593
              tunnel: [w652] -> w592
              tunnel: w443 -> [w697]
              tunnel: [w664] -> w591
              tunnel: w599 -> [w704]
              tunnel: [w672] -> w598
              tunnel: w543 -> [w702]
              tunnel: w530 -> [w674]
              tunnel: [w674] -> w540
              tunnel: w530 -> [w701]
              tunnel: w529 -> [w699]
              tunnel: [w698] -> w528
              tunnel: [w660] -> w523
              tunnel: [w659] -> w522
              tunnel: [w658] -> w521
              tunnel: [w663] -> w511
              tunnel: [w661] -> w510
              tunnel: w504 -> [w696]
              tunnel: [w696] -> w503
              tunnel: w502 -> [w695]
              tunnel: [w662] -> w489
              tunnel: [w657] -> w463
              tunnel: [w694] -> w451
              tunnel: w445 -> [w692]
              tunnel: [w676] -> w442
              tunnel: [w675] -> w434
              tunnel: w420 -> [w668]
              tunnel: w419 -> [w667]
              tunnel: [w667] -> w418
              tunnel: w414 -> [w666]
              tunnel: [w666] -> w413
              tunnel: w408 -> [w665]
              tunnel: [w665] -> w407
              tunnel: ["WS1050/51"] -> w400
              tunnel: ["Test Sequences"] -> w390
              tunnel: "Real No. From\nLookup Table" -> [w646]
              tunnel: ["Cmin/Act"] -> w386
              tunnel: w382 -> [w644]
              tunnel: w381 -> [w643]
              tunnel: w597 -> [w1024]
              tunnel: [w1020] -> w501
              tunnel: w596 -> [w1023]
              tunnel: w595 -> [w1030]
              tunnel: [w1030] -> w500
              tunnel: w594 -> [w1029]
              tunnel: w593 -> [w1022]
              tunnel: w592 -> [w1021]
              tunnel: [w1007] -> w499
              tunnel: [w1029] -> w498
              tunnel: [w1022] -> w497
              tunnel: [w1021] -> w496
              tunnel: w591 -> [w1027]
              tunnel: w540 -> [w1026]
              tunnel: [w1026] -> w495
              tunnel: w528 -> [w1025]
              tunnel: [w1025] -> w494
              tunnel: [w1023] -> w493
              tunnel: w523 -> [w1018]
              tunnel: w522 -> [w1012]
              tunnel: w521 -> [w1010]
              tunnel: [w1015] -> w492
              tunnel: w511 -> [w1017]
              tunnel: w510 -> [w1015]
              tunnel: [w1008] -> w491
              tunnel: w503 -> [w1016]
              tunnel: [w1013] -> w490
              tunnel: w489 -> [w1013]
              tunnel: [w1012] -> w488
              tunnel: w463 -> [w1011]
              tunnel: [w1011] -> w462
              tunnel: [w1010] -> w460
              tunnel: w451 -> [w1014]
              tunnel: [w1009] -> w435
              tunnel: w434 -> [w1009]
              tunnel: w418 -> [w1006]
              tunnel: [w1006] -> w417
              tunnel: w413 -> [w1005]
              tunnel: [w1005] -> w412
              tunnel: w407 -> [w1004]
              tunnel: [w1004] -> w406
              tunnel: w400 -> [w1000]
              tunnel: [w1000] -> w399
              tunnel: w390 -> [w999]
              tunnel: [w999] -> w389
              tunnel: w386 -> [w998]
              tunnel: [w998] -> w385
              tunnel: w501 -> [w1135]
              tunnel: [w1134] -> w487
              tunnel: w500 -> [w1148]
              tunnel: [w1148] -> w484
              tunnel: w499 -> [w1147]
              tunnel: [w1147] -> w482
              tunnel: w498 -> [w1146]
              tunnel: [w1146] -> w480
              tunnel: w497 -> [w1145]
              tunnel: [w1145] -> w478
              tunnel: w496 -> [w1144]
              tunnel: [w1144] -> w476
              tunnel: w495 -> [w1143]
              tunnel: [w1143] -> w474
              tunnel: w494 -> [w1142]
              tunnel: [w1142] -> w472
              tunnel: w493 -> [w1141]
              tunnel: [w1141] -> w470
              tunnel: w492 -> [w1140]
              tunnel: [w1140] -> w468
              tunnel: [w1129] -> w466
              tunnel: w491 -> [w1128]
              tunnel: w490 -> [w1138]
              tunnel: w488 -> [w1136]
              tunnel: w462 -> [w1133]
              tunnel: [w1133] -> w461
              tunnel: w460 -> [w1132]
              tunnel: [w1132] -> w459
              tunnel: [w1130] -> w458
              tunnel: [w1131] -> w436
              tunnel: w435 -> [w1131]
              tunnel: w417 -> [w1127]
              tunnel: [w1127] -> w416
              tunnel: w412 -> [w1126]
              tunnel: [w1126] -> w411
              tunnel: w406 -> [w1125]
              tunnel: [w1125] -> w405
              tunnel: w399 -> [w1124]
              tunnel: [w1124] -> w398
              tunnel: w389 -> [w1123]
              tunnel: [w1123] -> w388
              tunnel: w385 -> [w1122]
              tunnel: [w1122] -> w384
              tunnel: w487 -> [w1222]
              tunnel: [w1221] -> w486
              tunnel: [w1217] -> w485
              tunnel: w484 -> [w1234]
              tunnel: [w1234] -> w483
              tunnel: w482 -> [w1233]
              tunnel: [w1233] -> w481
              tunnel: w480 -> [w1232]
              tunnel: [w1232] -> w479
              tunnel: w478 -> [w1231]
              tunnel: [w1231] -> w477
              tunnel: w476 -> [w1230]
              tunnel: [w1230] -> w475
              tunnel: w474 -> [w1229]
              tunnel: [w1229] -> w473
              tunnel: w472 -> [w1228]
              tunnel: [w1228] -> w471
              tunnel: w470 -> [w1227]
              tunnel: [w1227] -> w469
              tunnel: w468 -> [w1226]
              tunnel: [w1226] -> w467
              tunnel: w466 -> [w1225]
              tunnel: [w1225] -> w465
              tunnel: [w1215] -> w464
              tunnel: w461 -> [w1224]
              tunnel: w459 -> [w1223]
              tunnel: w458 -> [w1216]
              tunnel: [w1220] -> w449
              tunnel: [w1219] -> w437
              tunnel: w436 -> [w1219]
              tunnel: w428 -> [w1218]
              tunnel: [w1218] -> w427
              tunnel: w416 -> [w1214]
              tunnel: [w1214] -> w415
              tunnel: w411 -> [w1213]
              tunnel: [w1213] -> w410
              tunnel: w405 -> [w1212]
              tunnel: [w1212] -> w404
              tunnel: w398 -> [w1211]
              tunnel: [w1211] -> w397
              tunnel: [w1211] -> w395
              tunnel: [w1211] -> w394
              tunnel: w388 -> [w1210]
              tunnel: w384 -> [w1209]
              tunnel: [w1209] -> w383
              tunnel: [w1362] -> w590
              tunnel: [w1328] -> w589
              tunnel: w486 -> [w1366]
              tunnel: w485 -> [w1342]
              tunnel: [w1351] -> w588
              tunnel: [w1342] -> w587
              tunnel: [w1365] -> w586
              tunnel: [w1364] -> w585
              tunnel: w483 -> [w1363]
              tunnel: [w1363] -> w584
              tunnel: w481 -> [w1351]
              tunnel: w479 -> [w1361]
              tunnel: [w1361] -> w583
              tunnel: w477 -> [w1357]
              tunnel: [w1357] -> w582
              tunnel: w475 -> [w1356]
              tunnel: [w1356] -> w581
              tunnel: w473 -> [w1352]
              tunnel: [w1352] -> w539
              tunnel: w471 -> [w1360]
              tunnel: [w1360] -> w527
              tunnel: w469 -> [w1359]
              tunnel: [w1358] -> w524
              tunnel: w467 -> [w1354]
              tunnel: w465 -> [w1350]
              tunnel: [w1355] -> w520
              tunnel: [w1353] -> w519
              tunnel: [w1350] -> w514
              tunnel: w464 -> [w1349]
              tunnel: [w1336] -> w509
              tunnel: [w1335] -> w508
              tunnel: [w1334] -> w507
              tunnel: w449 -> [w1348]
              tunnel: [w1333] -> w438
              tunnel: w437 -> [w1333]
              tunnel: [w1332] -> w433
              tunnel: w427 -> [w1331]
              tunnel: w415 -> [w1326]
              tunnel: w410 -> [w1325]
              tunnel: [w1325] -> w409
              tunnel: w404 -> [w1324]
              tunnel: [w1324] -> w403
              tunnel: w397 -> [w1314]
              tunnel: [w1314] -> w396
              tunnel: w395 -> [w1313]
              tunnel: w394 -> [w1312]
              tunnel: w383 -> [w1311]
              tunnel: w590 -> [w1585]
              tunnel: [w1585] -> w580
              tunnel: [w1570] -> w579
              tunnel: [w1584] -> w578
              tunnel: w589 -> [w1583]
              tunnel: w588 -> [w1582]
              tunnel: w587 -> [w1581]
              tunnel: [w1582] -> w577
              tunnel: [w1581] -> w576
              tunnel: w586 -> [w1580]
              tunnel: [w1580] -> w575
              tunnel: w585 -> [w1579]
              tunnel: [w1579] -> w574
              tunnel: w584 -> [w1578]
              tunnel: [w1578] -> w573
              tunnel: w583 -> [w1577]
              tunnel: [w1577] -> w572
              tunnel: w582 -> [w1576]
              tunnel: [w1576] -> w571
              tunnel: w581 -> [w1575]
              tunnel: [w1575] -> w570
              tunnel: w601 -> [w1574]
              tunnel: [w1572] -> w569
              tunnel: [w1552] -> w568
              tunnel: [w1553] -> w567
              tunnel: [w1551] -> w566
              tunnel: w539 -> [w1568]
              tunnel: [w1568] -> w538
              tunnel: w527 -> [w1567]
              tunnel: [w1567] -> w526
              tunnel: w524 -> [w1584]
              tunnel: w520 -> [w1565]
              tunnel: w519 -> [w1566]
              tunnel: [w1566] -> w518
              tunnel: [w1565] -> w516
              tunnel: w514 -> [w1564]
              tunnel: [w1564] -> w513
              tunnel: w509 -> [w1550]
              tunnel: w508 -> [w1549]
              tunnel: w507 -> [w1548]
              tunnel: [w1545] -> w506
              tunnel: [w1550] -> w457
              tunnel: [w1549] -> w455
              tunnel: [w1548] -> w453
              tunnel: [w1547] -> w439
              tunnel: w438 -> [w1547]
              tunnel: w433 -> [w1546]
              tunnel: [w1546] -> w432
              tunnel: w409 -> [w1545]
              tunnel: w403 -> [w1544]
              tunnel: w396 -> [w1543]
              tunnel: [w1543] -> w393
              tunnel: w580 -> [w1679]
              tunnel: [w1679] -> w565
              tunnel: w579 -> [w1703]
              tunnel: [w1702] -> w564
              tunnel: w617 -> [w1704]
              tunnel: w616 -> [w1701]
              tunnel: w615 -> [w1700]
              tunnel: w614 -> [w1699]
              tunnel: [w1698] -> w563
              tunnel: w578 -> [w1692]
              tunnel: [w1692] -> w562
              tunnel: w577 -> [w1697]
              tunnel: w576 -> [w1696]
              tunnel: [w1697] -> w561
              tunnel: [w1696] -> w560
              tunnel: [w1687] -> w559
              tunnel: w575 -> [w1695]
              tunnel: [w1695] -> w558
              tunnel: w574 -> [w1694]
              tunnel: [w1694] -> w557
              tunnel: w573 -> [w1691]
              tunnel: [w1693] -> w556
              tunnel: w426 -> [w1690]
              tunnel: [w1689] -> w555
              tunnel: [w1677] -> w554
              tunnel: w572 -> [w1688]
              tunnel: w571 -> [w1686]
              tunnel: w570 -> [w1685]
              tunnel: "File Name" -> [w1684]
              tunnel: w569 -> [w1683]
              tunnel: [w1683] -> w553
              tunnel: w568 -> [w1682]
              tunnel: [w1682] -> w552
              tunnel: [w1681] -> w551
              tunnel: w567 -> [w1681]
              tunnel: w566 -> [w1680]
              tunnel: [w1680] -> w550
              tunnel: [w1675] -> w541
              tunnel: w538 -> [w1676]
              tunnel: [w1676] -> w536
              tunnel: w533 -> [w1674]
              tunnel: w526 -> [w1673]
              tunnel: [w1673] -> w525
              tunnel: w518 -> [w1672]
              tunnel: [w1672] -> w517
              tunnel: w516 -> [w1671]
              tunnel: [w1671] -> w515
              tunnel: w513 -> [w1670]
              tunnel: [w1670] -> w512
              tunnel: w506 -> [w1669]
              tunnel: w457 -> [w1668]
              tunnel: [w1668] -> w456
              tunnel: w455 -> [w1667]
              tunnel: [w1667] -> w454
              tunnel: w453 -> [w1666]
              tunnel: [w1666] -> w452
              tunnel: w442 -> [w1665]
              tunnel: [w1665] -> w441
              tunnel: [w1664] -> w440
              tunnel: w439 -> [w1664]
              tunnel: w432 -> [w1663]
              tunnel: [w1663] -> w431
              tunnel: ["Freq(Hz)"] -> w402
              tunnel: ["Brd #"] -> w401
              tunnel: w393 -> [w1660]
              tunnel: [w1660] -> w392
              tunnel: w565 -> [w1775]
              tunnel: w564 -> [w1774]
              tunnel: w617 -> [w1736]
              tunnel: w613 -> [w1769]
              tunnel: w612 -> [w1772]
              tunnel: w611 -> [w1768]
              tunnel: w610 -> [w1771]
              tunnel: w609 -> [w1767]
              tunnel: w563 -> [w1770]
              tunnel: [w1775] -> w546
              tunnel: [w1773] -> w547
              tunnel: w562 -> [w1765]
              tunnel: [w1765] -> w548
              tunnel: w561 -> [w1764]
              tunnel: w560 -> [w1749]
              tunnel: w559 -> [w1763]
              tunnel: w558 -> [w1762]
              tunnel: w557 -> [w1751]
              tunnel: [w1759] -> w549
              tunnel: w556 -> [w1761]
              tunnel: w555 -> [w1760]
              tunnel: w554 -> [w1759]
              tunnel: "File Name" -> [w1729]
              tunnel: w553 -> [w1758]
              tunnel: [w1758] -> w545
              tunnel: w552 -> [w1757]
              tunnel: w551 -> [w1756]
              tunnel: w550 -> [w1755]
              tunnel: [w1754] -> w542
              tunnel: w541 -> [w1754]
              tunnel: [w1732] -> w537
              tunnel: w536 -> [w1732]
              tunnel: w525 -> [w1753]
              tunnel: w517 -> [w1752]
              tunnel: w515 -> [w1750]
              tunnel: w512 -> [w1748]
              tunnel: w456 -> [w1747]
              tunnel: w454 -> [w1746]
              tunnel: w452 -> [w1745]
              tunnel: w450 -> [w1744]
              tunnel: w430 -> [w1742]
              tunnel: w444 -> [w1741]
              tunnel: w448 -> [w1740]
              tunnel: w441 -> [w1739]
              tunnel: w440 -> [w1738]
              tunnel: w431 -> [w1737]
              tunnel: [w1734] -> w425
              tunnel: [w1725] -> w421
              tunnel: w402 -> [w1724]
              tunnel: w401 -> [w1723]
              tunnel: w392 -> [w1722]
              tunnel: [w1722] -> w391
              tunnel: [w1797] -> w607
              tunnel: [w1798] -> w608
              tunnel: [w1799] -> w505
              tunnel: w549 -> [w1790]
              tunnel: w548 -> [w1798]
              tunnel: w547 -> [w1785]
              tunnel: w546 -> [w1799]
              tunnel: w545 -> [w1792]
              tunnel: [w1792] -> w600
              tunnel: [w1789] -> w534
              tunnel: w542 -> [w1789]
              tunnel: w537 -> [w1791]
              tunnel: [w1791] -> w535
              tunnel: [w1790] -> w532
              tunnel: [w1788] -> w531
              tunnel: [w1784] -> w422
              tunnel: w425 -> [w1783]
              tunnel: w421 -> [w1781]
              tunnel: w391 -> [w1780]
              frame #0 {
                n128 = call "WSVCAP SHL Host TL RFFE Write - Multiple DUTs - Common Data.vi"("Data Out"=w692, "error in"=w697) -> ("error out"=w670:errorcluster)  [unwired: 13 in]
                n129 = Index Array(array=w708, index (row)=w701, index (col)=0 ("disabled index (col)")) -> (element=w700:dbl)
                n130 = for {
                  tunnel: string[] ["0760", "0767", "0768"] -> [w755] mode=indexing
                  tunnel: [w751] -> w681 mode=indexing
                  tunnel: w670 -> [w749]
                  tunnel: [w748] -> w673
                  i -> [w754]
                  n131 = call "Delay T4.vi"("milliseconds to wait"=u32 10, "error in (no error)"=w749) -> ("error out"=w756:errorcluster)  [unwired: 9 in]
                  n132 = call "WSVCAP SHL Host TL RFFE Read - Multiple DUTs - Common Data.vi"("Data Out"=w755, "error in"=w756) -> ("RFFE Data In"=w753:string[], "error out"=w748:errorcluster)  [unwired: 12 in]
                  n133 = Index Array(array=w753, index=w754) -> (element=w750:string)
                  n134 = String Subset(string=w750, offset (0)=0) -> (substring=w751:string)  [unwired: 1 in]
                }
                "RB Reg for HD/Cycle" <- w681
                n135 = call "Delay T4.vi"("milliseconds to wait"=u32 100, "error in (no error)"=w673) -> ("error out"=w687:errorcluster)  [unwired: 9 in]
                n136 = local read "IDD Brd(uA)"() -> (w691:string)
                n137 = call "Ke2000 Reading MilAmp.vi"("error in (no error)"=w687, "VISA resource name"=w684) -> ("error out"=w689:errorcluster, "uA"=w690:string, "VISA resource name out"=w683:refnum<visa-resource-name>)  [unwired: 7 in]
                n138 = call "Substration.vi"("error in (no error)"=w689, "Input2"=w691, "Input1"=w690) -> ("error out"=w686:errorcluster, "In1 - In2"=→"IDD_HD/CYC (uA)":string)  [unwired: 7 in]
                n139 = case shown="True" w699 {
                  tunnel: [w788 w885] -> w710
                  tunnel: [w789 w870] -> w705
                  tunnel: [w787 w887] -> w707
                  tunnel: w686 -> [w783 w874]
                  tunnel: w704 -> [w779 w886]
                  tunnel: [w779 w886] -> w672
                  tunnel: w702 -> [_ w876]
                  tunnel: w700 -> [w780 w871]
                  tunnel: [w785 w872] -> w698
                  tunnel: w674 -> [w771 w868]
                  tunnel: w695 -> [w782 _]
                  tunnel: ["%Duty Cycle" "100" ("Data Out")] -> w676
                  tunnel: w668 -> [w769 _]
                  tunnel: w646 -> [w768 w861]
                  tunnel: w644 -> [w765 _]
                  tunnel: w643 -> [w764 _]
                  frame False {
                    # "Cycles in 1s"
                    n140 = case shown="False" w768 {
                      tunnel: w783 -> [w795 w801]
                      tunnel: w780 -> [w794 w800]
                      tunnel: [w793 w801] -> w778
                      tunnel: w771 -> [w792 _]
                      tunnel: [w791 w800] -> w777
                      tunnel: [u64 1000 ("y") u64 1 ("y")] -> w772
                      frame False {
                        n141 = case shown="8, Default" w792 {
                          tunnel: w794 -> [w797 _]
                          tunnel: [w797 "CYC RP (X1000)"] -> w791
                          tunnel: [w796 w798] -> w793
                          tunnel: w795 -> [w796 w798]
                          frame 0..7 {
                          }
                          frame 8, Default {
                          }
                        }
                      }
                      frame True {
                        # "Read real number\nfrom lookup table"
                      }
                    }
                    n142 = call "WSVCAP SHL Host TL RFFE Configure.vi"("RFFE Slave Address"=w782, "Clock Rate (Hz)"="SPI Clock Rate (Hz)", "error in"=w778) -> ("Actual Rate (Hz)"=→"AR Cycling(Hz)":dbl, "error out"=w766:errorcluster)  [unwired: 11 in]
                    n143 = Array Max & Min(array=w764) -> (max value=w775:dbl)  [unwired: 3 out]
                    n144 = Divide(x=1.0, y=w775) -> (x/y=w774:dbl)
                    n145 = To Unsigned Quad Integer(1:w774) -> (0:w773:u64)
                    n146 = Not(x=w769) -> (.not. x?=w770:bool)
                    n147 = case shown="True" w770 {
                      tunnel: [w804 w826] -> w789
                      tunnel: [w807 w825] -> w788
                      tunnel: [u64 1 w824] -> w787
                      tunnel: w766 -> [w805 w823]
                      tunnel: w777 -> [_ w822]
                      tunnel: w764 -> [_ w820]
                      tunnel: w773 -> [_ w819]
                      tunnel: w772 -> [_ w818]
                      tunnel: w771 -> [w803 _]
                      tunnel: w765 -> [_ w817]
                      frame False {
                        n148 = case shown="1, Default" w803 {
                          tunnel: w805 -> [w808 w810]
                          tunnel: [w808 w809] -> w804
                          frame 0 {
                          }
                          frame 1, Default {
                            n149 = flat-sequence {
                              tunnel: "Repeat Meas(s)" -> [w816]
                              tunnel: w810 -> [w813]
                              tunnel: [w813] -> w809
                              frame #0 {
                                n150 = Multiply(x=w816, y=u32 1000) -> (x*y=w815:u32)
                                n151 = Wait (ms)(milliseconds to wait=w815) -> ()  [unwired: 1 out]
                                n152 = local write "STATUS"("Verify Sockets waiting times..." ("STATUS")) -> ()
                              }
                            }
                          }
                        }
                        n153 = local read "stop During HD/Cycles"() -> (w807:bool)
                      }
                      frame True {
                        n154 = while {
                          tunnel: w822 -> [w846]
                          tunnel: [w833] -> w826
                          tunnel: [w838] -> w825
                          tunnel: w823 -> [w844]
                          tunnel: [w832] -> w824
                          tunnel: w817 -> [w843]
                          tunnel: w820 -> [w842]
                          tunnel: w819 -> [w829]
                          tunnel: w818 -> [w827]
                          i -> [w841]
                          stop <- w837 stop-if-true
                          # "At least 1 second before target"
                          # "Remaining Cycles"
                          # "Target Cycles"
                          # "Cycles in 1s"
                          n155 = To Unsigned Quad Integer(1:w846) -> (0:w845:u64)
                          n156 = case shown="0" w841 {
                            tunnel: [w853 w855] -> w835
                            tunnel: w844 -> [w854 w855]
                            tunnel: w843 -> [w852 _]
                            tunnel: w842 -> [w851 _]
                            frame 0 {
                              n157 = call "WSVCAP SHL Host TL RFFE Write Cycle - Multiple DUTs - Common Data1.vi"("Data Out (Cycle Commands)"=w852, "Post Command Delay"=w851, "error in"=w854) -> ("error out"=w853:errorcluster)  [unwired: 12 in]
                            }
                            frame 1, Default {
                            }
                          }
                          n158 = Multiply(x=w845, y=w827) -> (x*y=w832:u64)
                          n159 = call "WSVCAP SHL Host TL SPI_RFFE Query Cycle Count.vi"("error in"=w835) -> ("Cycle Count"=w831:u64, "error out"=w840:errorcluster)  [unwired: 13 in]
                          "Cycle Count" <- w831
                          n160 = Subtract(x=w832, y=w831) -> (x-y=w830:u64)
                          n161 = Greater Or Equal?(x=w831, y=w832) -> (x >= y?=w839:bool)
                          n162 = local read "stop During HD/Cycles"() -> (w838:bool)
                          n163 = Greater?(x=w830, y=w829) -> (0:w828:bool)
                          n164 = case shown="True" w839 {
                            tunnel: [w857 w860] -> w834
                            tunnel: w840 -> [w857 w859]
                            tunnel: [FALSE TRUE] -> w836
                            frame False {
                            }
                            frame True {
                              n165 = call "WSVCAP SHL Host TL RFFE Stop Write Cycle.vi"("error in"=w859) -> ("error out"=w860:errorcluster)  [unwired: 14 in]
                            }
                          }
                          n166 = Or(x=w836, y=w838) -> (x .or. y?=w837:bool)
                          n167 = case shown="True" w828 {
                            tunnel: w834 -> [w847 w850]
                            tunnel: [w847 w849] -> w833
                            frame False {
                            }
                            frame True {
                              n168 = call "MISC Wait with Data Flow.vi"("Error In (no error)"=w850, "Wait Time (500ms)"=u32 50) -> ("Error Out"=w849:errorcluster)  [unwired: 7 in, 2 out]
                            }
                          }
                        }
                        n169 = local write "STATUS"("Parts are Cycling...." ("STATUS")) -> ()
                      }
                    }
                    n170 = local read "HD/CYC Temp"() -> (w784:i32)
                    n171 = Number To Engineering String(4:w784) -> (0:w785:string)  [unwired: 3 in]
                  }
                  frame True {
                    n172 = case shown="False" w861 {
                      tunnel: w876 -> [w893 _]
                      tunnel: [w892 w905] -> w875
                      tunnel: w874 -> [w891 w906]
                      tunnel: [w890 w906] -> w873
                      tunnel: w871 -> [w889 w905]
                      tunnel: w868 -> [w888 _]
                      frame False {
                        n173 = case shown="0" w893 {
                          tunnel: [w896 w903] -> w892
                          tunnel: w891 -> [w898 w904]
                          tunnel: [w897 w904] -> w890
                          tunnel: w889 -> [w895 _]
                          tunnel: w888 -> [w894 _]
                          frame 0 {
                            n174 = case shown="15, Default" w894 {
                              tunnel: [w899 "HD RP(Min)"] -> w896
                              tunnel: w898 -> [w900 w902]
                              tunnel: [w900 w902] -> w897
                              tunnel: w895 -> [w899 _]
                              frame 0..14 {
                              }
                              frame 15, Default {
                              }
                            }
                          }
                          frame 1, Default {
                            n175 = local read "HD RP(Min)"() -> (w903:dbl)
                          }
                        }
                      }
                      frame True {
                      }
                    }
                    n176 = flat-sequence {
                      tunnel: [w980] -> w881
                      tunnel: w873 -> [w986]
                      frame #0 {
                        n177 = call "WSVCAP SHL Host TL RFFE Write - Multiple DUTs - Common Data.vi"("Data Out"="Cmd to HD", "error in"=w986) -> ("error out"=w985:errorcluster)  [unwired: 13 in]
                        n178 = call "Delay T4.vi"("milliseconds to wait"=u32 50, "error in (no error)"=w985) -> ("error out"=w982:errorcluster)  [unwired: 9 in]
                        n179 = for {
                          tunnel: string[] ["0761", "0762", "0763"] -> [w997] mode=indexing
                          tunnel: [w993] -> w981 mode=indexing
                          shift-right: [w990] -> w980
                          shift-left: w982 -> [w996]
                          i -> [w995]
                          n180 = call "WSVCAP SHL Host TL RFFE Read - Multiple DUTs - Common Data.vi"("Data Out"=w997, "error in"=w996) -> ("RFFE Data In"=w992:string[], "error out"=w989:errorcluster)  [unwired: 12 in]
                          n181 = Index Array(array=w992, index=w995) -> (element=w991:string)
                          n182 = call "Delay T4.vi"("milliseconds to wait"=u32 10, "error in (no error)"=w989) -> ("error out"=w990:errorcluster)  [unwired: 9 in]
                          n183 = String Subset(string=w991, offset (0)=0) -> (substring=w993:string)  [unwired: 1 in]
                        }
                        "RB Reg for HD" <- w981
                      }
                    }
                    n184 = local read "No of HD/Cycle\nCompleted"() -> (w877:u64)
                    n185 = Greater?(x="HD_DC (Min)", y=w877) -> (0:w878:bool)
                    n186 = case shown="True" w878 {
                      tunnel: [_ w913] -> w883
                      tunnel: [w908 w912] -> w882
                      tunnel: w881 -> [w908 w911]
                      tunnel: w875 -> [w907 w910]
                      tunnel: [w907 w909] -> w880
                      frame False {
                      }
                      frame True {
                        n187 = flat-sequence {
                          tunnel: [w918] -> w913
                          tunnel: [w917] -> w912
                          tunnel: w911 -> [w916]
                          tunnel: w910 -> [w914]
                          tunnel: [w914] -> w909
                          frame #0 {
                            # "HD"
                            n188 = Multiply(x=1000.0, y=w914) -> (x*y=w921:dbl)
                            n189 = Multiply(x=60.0, y=w921) -> (x*y=w919:dbl)
                            n190 = local write "STATUS"("Parts are Holding Down..." ("STATUS")) -> ()
                            n191 = event shown="[0] Timeout" {
                              selector: _ -> [_ _]
                              dyn-events: _ -> [_ _]
                              timeout: w919 -> [_ _]
                              tunnel: ["stop During HD/Cycles" TRUE ("stop During HD/Cycles")] -> w918
                              tunnel: w916 -> [w923 w925]
                              tunnel: [w923 w925] -> w917
                              event Timeout {
                                n192 = event-data() -> ()  [unwired: 1 in, 2 out]
                              }
                              event "stop During HD/Cycles": Value Change {
                                n193 = event-data() -> ()  [unwired: 1 in, 2 out]
                              }
                            }
                          }
                        }
                      }
                    }
                    n194 = Greater Or Equal?(x=w877, y="HD_DC (Min)") -> (x >= y?=w884:bool)
                    n195 = To Unsigned Quad Integer(1:w875) -> (0:w887:u64)
                    n196 = Add(x="Time All OFF (s)", y="Time All ON (s)") -> (x+y=w863:u32)
                    n197 = To Double Precision Float(number=w863) -> (double precision float=w862:dbl)
                    n198 = Divide(x=w862, y=60.0) -> (x/y=w864:dbl)
                    n199 = case shown="False" w884 {
                      tunnel: [w929 w942] -> w885
                      tunnel: [w930 w934] -> w870
                      tunnel: w882 -> [w930 w941]
                      tunnel: w883 -> [w929 w940]
                      tunnel: w880 -> [_ w939]
                      tunnel: [w928 w937] -> w872
                      tunnel: w864 -> [_ w931]
                      frame False {
                        n200 = Number To Engineering String(4:"HD/CYC Temp") -> (0:w928:string)  [unwired: 3 in]
                      }
                      frame True {
                        n201 = Divide(x=w939, y=w931) -> (x/y=w938:dbl)
                        n202 = call "WSVCAP SHL Host TL RFFE Write - Multiple DUTs - Common Data.vi"("Data Out"="070201000000", "error in"=w941) -> ("error out"=w944:errorcluster)  [unwired: 13 in]
                        n203 = Round To Nearest(number=w938) -> (nearest integer value=w933:dbl)
                        n204 = call "Delay T4.vi"("milliseconds to wait"=u32 50, "error in (no error)"=w944) -> ("error out"=w935:errorcluster)  [unwired: 9 in]
                        n205 = To Long Integer(number=w933) -> (32bit integer=w932:i32)
                        "No LPs to RP" <- w932
                        n206 = for {
                          N: w932 -> [_]
                          tunnel: w940 -> [w959]
                          tunnel: [w958] -> w942
                          tunnel: w935 -> [w947]
                          tunnel: [w946] -> w934
                          i -> [w957]
                          stop <- w958 stop-if-true
                          n207 = Increment(x=w957) -> (x+1=→"LPs Count":i32)
                          n208 = call "WSVCAP SHL Host TL RFFE Write - Multiple DUTs - Common Data.vi"("Data Out"="074776", "error in"=w947) -> ("error out"=w965:errorcluster)  [unwired: 13 in]
                          n209 = call "Delay T4.vi"("milliseconds to wait"=u32 1, "error in (no error)"=w965) -> ("error out"=w964:errorcluster)  [unwired: 9 in]
                          n210 = local read "CP to HD/Cycle"() -> (w949:i32)
                          n211 = call "WSVCAP SHL Host TL RFFE Write - Multiple DUTs - Common Data.vi"("Data Out"="070201000000", "error in"=w950) -> ("error out"=w961:errorcluster)  [unwired: 13 in]
                          n212 = call "WSVCAP SHL Host TL RFFE Write - Multiple DUTs - Common Data.vi"("Data Out"="0702013B3B3B", "error in"=w964) -> ("error out"=w954:errorcluster)  [unwired: 13 in]
                          n213 = flat-sequence {
                            tunnel: w961 -> [w973]
                            tunnel: [w971] -> w946
                            frame #0 {
                              n214 = local read "Time All OFF (s)"() -> (w968:u32)
                              n215 = local write "STATUS"("Now HD OFF Time..." ("STATUS")) -> ()
                              n216 = Multiply(x=w968, y=u32 1000) -> (x*y=w970:u32)
                              n217 = call "Delay T4.vi"("milliseconds to wait"=w970, "error in (no error)"=w973) -> ("error out"=w971:errorcluster)  [unwired: 9 in]
                            }
                          }
                          n218 = call "Delay T4.vi"("milliseconds to wait"=u32 1, "error in (no error)"=w954) -> ("error out"=w952:errorcluster)  [unwired: 9 in]
                          n219 = Index Array(array=string[] ["07476F", "074776", "074765", "074769", "07477B"], index=w949) -> (element=w955:string)
                          n220 = call "WSVCAP SHL Host TL RFFE Write - Multiple DUTs - Common Data.vi"("Data Out"=w955, "error in"=w952) -> ("error out"=w951:errorcluster)  [unwired: 13 in]
                          n221 = flat-sequence {
                            tunnel: [w978] -> w950
                            tunnel: w951 -> [w974]
                            frame #0 {
                              n222 = local read "Time All ON (s)"() -> (w975:u32)
                              n223 = local write "STATUS"("Now HD ON Time..." ("STATUS")) -> ()
                              n224 = Multiply(x=w975, y=u32 1000) -> (x*y=w977:u32)
                              n225 = call "Delay T4.vi"("milliseconds to wait"=w977, "error in (no error)"=w974) -> ("error out"=w978:errorcluster)  [unwired: 9 in]
                            }
                          }
                          n226 = Unbundle By Name(w946) -> ("status"=w960:bool)
                          n227 = Or(x=w960, y=w959) -> (x .or. y?=w958:bool)
                        }
                        n228 = Number To Engineering String(4:"DC_Temp") -> (0:w937:string)  [unwired: 3 in]
                      }
                    }
                  }
                }
                n229 = case shown="4" "CP to Meas" {
                  selector: "CP to Meas" -> [w726 w731 w736 w741 w745]
                  tunnel: string[] ["07476F", "074776", "074765", "074769", "07477B"] -> [w727 w732 w737 w742 w747]
                  tunnel: [w725 w730 w735 w740 w746] -> w679
                  tunnel: [w724 w729 w734 w739 w744] -> w669
                  tunnel: w678 -> [w724 w729 w734 w739 w744]
                  tunnel: ["35" ("Data Out") "27.5" ("Data Out") "30.5" ("Data Out") "44.0" ("Data Out") "40.25" ("Data Out")] -> w675
                  frame 0, Default {
                    n230 = Index Array(array=w727, index=w726) -> (element=w725:string)
                  }
                  frame 2 {
                    n231 = Index Array(array=w732, index=w731) -> (element=w730:string)
                  }
                  frame 3 {
                    n232 = Index Array(array=w737, index=w736) -> (element=w735:string)
                  }
                  frame 4 {
                    n233 = Index Array(array=w742, index=w741) -> (element=w740:string)
                  }
                  frame 1 {
                    n234 = Index Array(array=w747, index=w745) -> (element=w746:string)
                  }
                }
                n235 = call "WSVCAP SHL Host TL RFFE Write - Multiple DUTs - Common Data.vi"("Data Out"=w679, "error in"=w669) -> ("error out"=w693:errorcluster)  [unwired: 13 in]
                n236 = flat-sequence {
                  tunnel: w705 -> [w763]
                  tunnel: [w763] -> w678
                  frame #0 {
                    w759 = "0" ("NOM IDD OFF(uA)")
                    w760 = string[] []
                    w761 = string[][] []
                    n237 = To Long Integer(number=0.0 ("No of Loops to RP")) -> (32bit integer=w758:i32)
                    n238 = local write "LPs Count"(w758) -> ()
                    n239 = local write "No LPs to RP"(w758) -> ()
                    n240 = local write "NOM IDD ON (uA)"(w759) -> ()
                    n241 = local write "Current EFuse Read back"(w760) -> ()
                    n242 = local write "RB Reg for HD"(w760) -> ()
                    n243 = local write "RB Reg for HD/Cycle"(w760) -> ()
                    n244 = local write "NOM IDD OFF(uA)"(w759) -> ()
                    n245 = local write "Total Delta 1(pF)"(w760) -> ()
                    n246 = local write "Total Delta 2(pF)"(w760) -> ()
                    n247 = local write "Total Delta 3(pF)"(w760) -> ()
                    n248 = local write "VSA_V3"(w761) -> ()
                    n249 = local write "VSA_V1"(w761) -> ()
                    n250 = local write "VSA_V2"(w761) -> ()
                    n251 = local write "VPI C1"(w761) -> ()
                    n252 = local write "VPI C2"(w761) -> ()
                    n253 = local write "VPI C3"(w761) -> ()
                    n254 = local write "% Delta C"(w761) -> ()
                    n255 = local write "40V_3"(w761) -> ()
                    n256 = local write "40V_2"(w761) -> ()
                    n257 = local write "40V_1"(w761) -> ()
                  }
                }
                n258 = call "Delay T4.vi"("milliseconds to wait"=u32 50, "error in (no error)"=w693) -> ("error out"=w671:errorcluster)  [unwired: 9 in]
                n259 = for {
                  tunnel: [w722] -> w650 mode=indexing
                  tunnel: w683 -> [w720]
                  tunnel: w671 -> [w719]
                  tunnel: [w713] -> w655
                  tunnel: string[] ["0702013B3B3B", "070201000000"] -> [w712] mode=indexing
                  tunnel: [w711] -> w648
                  n260 = call "WSVCAP SHL Host TL RFFE Write - Multiple DUTs - Common Data.vi"("Data Out"=w712, "error in"=w719) -> ("error out"=w716:errorcluster)  [unwired: 13 in]
                  n261 = call "Delay T4.vi"("milliseconds to wait"=u32 100, "error in (no error)"=w716) -> ("error out"=w717:errorcluster)  [unwired: 9 in]
                  n262 = local read "IDD Brd(uA)"() -> (w721:string)
                  n263 = call "Ke2000 Reading MilAmp.vi"("error in (no error)"=w717, "VISA resource name"=w720) -> ("error out"=w715:errorcluster, "uA"=w714:string, "VISA resource name out"=w713:refnum<visa-resource-name>)  [unwired: 7 in]
                  n264 = call "Substration.vi"("error in (no error)"=w715, "Input2"=w721, "Input1"=w714) -> ("error out"=w711:errorcluster, "In1 - In2"=w722:string)  [unwired: 7 in]
                }
                n265 = Index Array(array=w650, index=0) -> (element=w652:string)
                n266 = Index Array(array=w650, index=1) -> (element=w649:string)
                n267 = call "Multi Dut Cmd Setting.vi"("error in (no error)"=w648, "Test Seq"="Test Sequences", "Cmin/Act"="Cmin/Act", "WS1050/51"="WS1050/51") -> ("error out"=w664:errorcluster, "Cmd 3"=w658:string[], "Name 3"=w657:string[], "Name Header"=w661:string[], "Cmd 2"=w659:string[], "Name 2"=w662:string[], "Cmd 1"=w660:string[], "Name 1"=w663:string[])
                n268 = local read "SPI Clock Rate (Hz)"() -> (w694:dbl)
              }
              frame #1 {
                n269 = call "WSVCAP SHL Host TL RFFE Configure.vi"("RFFE Slave Address"=w1016, "Clock Rate (Hz)"=w1014, "error in"=w1027) -> ("Actual Rate (Hz)"=w1028:dbl, "error out"=w1002:errorcluster)  [unwired: 11 in]
                n270 = local write "AR  Meas(Hz)"(w1028) -> ()
                n271 = Array Size(array=w1017) -> (size(s)=w1031:i32)
                n272 = call "Delay T4.vi"("milliseconds to wait"=u32 10, "error in (no error)"=w1002) -> ("error out"=w1003:errorcluster)  [unwired: 9 in]
                n273 = case shown="2" w999 {
                  tunnel: w1031 -> [w1039 w1069 w1099]
                  tunnel: w1024 -> [w1038 w1068 w1098]
                  tunnel: [w1037 w1067 w1097] -> w1020
                  tunnel: [w1036 w1066 w1096] -> w1019
                  tunnel: w1018 -> [w1035 w1065 w1095]
                  tunnel: w1017 -> [w1034 w1064 w1094]
                  tunnel: [w1033 w1063 w1093] -> w1008
                  tunnel: w1003 -> [w1032 w1062 w1092]
                  frame 0, Default {
                    n274 = for {
                      N: w1039 -> [_]
                      tunnel: w1035 -> [w1057]
                      tunnel: w1038 -> [w1055]
                      tunnel: [w1054] -> w1037
                      tunnel: [w1050] -> w1036 mode=indexing
                      tunnel: w1034 -> [w1052]
                      tunnel: w1032 -> [w1040]
                      tunnel: [w1042] -> w1033
                      i -> [w1049]
                      stop <- w1054 stop-if-true
                      n275 = Index Array(array=w1057, index=w1049) -> (element=w1053:string)
                      n276 = Index Array(array=w1052, index=w1049) -> (element=w1051:string)
                      n277 = local write "STATUS"(w1051) -> ()
                      n278 = call "WSVCAP SHL Host TL RFFE Write - Multiple DUTs - Common Data.vi"("Data Out"=w1053, "error in"=w1040) -> ("error out"=w1044:errorcluster)  [unwired: 13 in]
                      n279 = call "Delay T4.vi"("milliseconds to wait"=u32 10, "error in (no error)"=w1044) -> ("error out"=w1048:errorcluster)  [unwired: 9 in]
                      n280 = call "WS1050 AD7747 READ.vi"("error in"=w1048, "Log (T)"=FALSE, "DUT Mask Mode (All)"=WSVCAP_SHL_I2C_DUT_Mask_Mode_Enum."C1") -> ("error out"=w1046:errorcluster, "AD7747 Values"=w1047:string[][])  [unwired: 7 in]
                      n281 = for {
                        tunnel: w1047 -> [w1060] mode=indexing
                        tunnel: w1046 -> [w1061]
                        tunnel: [w1061] -> w1042
                        tunnel: [w1058] -> w1050 mode=indexing
                        n282 = Index Array(array=w1060, index=1) -> (element=w1058:string)
                      }
                      n283 = Unbundle By Name(w1042) -> ("status"=w1056:bool)
                      n284 = Or(x=w1056, y=w1055) -> (x .or. y?=w1054:bool)
                    }
                  }
                  frame 1 {
                    n285 = for {
                      N: w1069 -> [_]
                      tunnel: w1065 -> [w1087]
                      tunnel: w1068 -> [w1085]
                      tunnel: [w1084] -> w1067
                      tunnel: [w1080] -> w1066 mode=indexing
                      tunnel: w1064 -> [w1082]
                      tunnel: w1062 -> [w1070]
                      tunnel: [w1072] -> w1063
                      i -> [w1079]
                      stop <- w1084 stop-if-true
                      n286 = Index Array(array=w1087, index=w1079) -> (element=w1083:string)
                      n287 = Index Array(array=w1082, index=w1079) -> (element=w1081:string)
                      n288 = local write "STATUS"(w1081) -> ()
                      n289 = call "WSVCAP SHL Host TL RFFE Write - Multiple DUTs - Common Data.vi"("Data Out"=w1083, "error in"=w1070) -> ("error out"=w1074:errorcluster)  [unwired: 13 in]
                      n290 = call "Delay T4.vi"("milliseconds to wait"=u32 10, "error in (no error)"=w1074) -> ("error out"=w1078:errorcluster)  [unwired: 9 in]
                      n291 = call "WS1050 AD7747 READ.vi"("error in"=w1078, "Log (T)"=FALSE, "DUT Mask Mode (All)"=WSVCAP_SHL_I2C_DUT_Mask_Mode_Enum."C2") -> ("error out"=w1076:errorcluster, "AD7747 Values"=w1077:string[][])  [unwired: 7 in]
                      n292 = for {
                        tunnel: w1077 -> [w1090] mode=indexing
                        tunnel: w1076 -> [w1091]
                        tunnel: [w1091] -> w1072
                        tunnel: [w1088] -> w1080 mode=indexing
                        n293 = Index Array(array=w1090, index=3) -> (element=w1088:string)
                      }
                      n294 = Unbundle By Name(w1072) -> ("status"=w1086:bool)
                      n295 = Or(x=w1086, y=w1085) -> (x .or. y?=w1084:bool)
                    }
                  }
                  frame 2 {
                    n296 = for {
                      N: w1099 -> [_]
                      tunnel: w1095 -> [w1117]
                      tunnel: w1098 -> [w1115]
                      tunnel: [w1114] -> w1097
                      tunnel: [w1110] -> w1096 mode=indexing
                      tunnel: w1094 -> [w1112]
                      tunnel: w1092 -> [w1100]
                      tunnel: [w1102] -> w1093
                      i -> [w1109]
                      stop <- w1114 stop-if-true
                      n297 = Index Array(array=w1117, index=w1109) -> (element=w1113:string)
                      n298 = Index Array(array=w1112, index=w1109) -> (element=w1111:string)
                      n299 = local write "STATUS"(w1111) -> ()
                      n300 = call "WSVCAP SHL Host TL RFFE Write - Multiple DUTs - Common Data.vi"("Data Out"=w1113, "error in"=w1100) -> ("error out"=w1104:errorcluster)  [unwired: 13 in]
                      n301 = call "Delay T4.vi"("milliseconds to wait"=u32 10, "error in (no error)"=w1104) -> ("error out"=w1108:errorcluster)  [unwired: 9 in]
                      n302 = call "WS1050 AD7747 READ.vi"("error in"=w1108, "Log (T)"=FALSE, "DUT Mask Mode (All)"=WSVCAP_SHL_I2C_DUT_Mask_Mode_Enum."C3") -> ("error out"=w1106:errorcluster, "AD7747 Values"=w1107:string[][])  [unwired: 7 in]
                      n303 = for {
                        tunnel: w1107 -> [w1120] mode=indexing
                        tunnel: w1106 -> [w1121]
                        tunnel: [w1121] -> w1102
                        tunnel: [w1118] -> w1110 mode=indexing
                        n304 = Index Array(array=w1120, index=5) -> (element=w1118:string)
                      }
                      n305 = Unbundle By Name(w1102) -> ("status"=w1116:bool)
                      n306 = Or(x=w1116, y=w1115) -> (x .or. y?=w1114:bool)
                    }
                  }
                }
                n307 = Transpose 2D Array(2D array=w1019) -> (transposed array=w1007:string[][])
                "40V_1" <- w1007
                "NOM IDD ON (uA)" <- w1022
                "NOM IDD OFF(uA)" <- w1021
              }
              frame #2 {
                n308 = Array Size(array=w1138) -> (size(s)=w1139:i32)
                n309 = case shown="0, 2, Default" w1123 {
                  tunnel: w1139 -> [w1156 w1186]
                  tunnel: w1138 -> [w1155 w1185]
                  tunnel: [w1154 w1184] -> w1137
                  tunnel: w1136 -> [w1153 w1183]
                  tunnel: w1135 -> [w1152 w1182]
                  tunnel: [w1151 w1181] -> w1134
                  tunnel: [w1150 w1180] -> w1130
                  tunnel: w1128 -> [w1149 w1179]
                  frame 0, 2, Default {
                    n310 = for {
                      N: w1156 -> [_]
                      tunnel: w1153 -> [w1174]
                      tunnel: w1152 -> [w1172]
                      tunnel: [w1171] -> w1151
                      tunnel: [w1167] -> w1154 mode=indexing
                      tunnel: w1155 -> [w1169]
                      tunnel: w1149 -> [w1157]
                      tunnel: [w1159] -> w1150
                      i -> [w1166]
                      stop <- w1171 stop-if-true
                      n311 = Index Array(array=w1174, index=w1166) -> (element=w1170:string)
                      n312 = Index Array(array=w1169, index=w1166) -> (element=w1168:string)
                      n313 = call "WSVCAP SHL Host TL RFFE Write - Multiple DUTs - Common Data.vi"("Data Out"=w1170, "error in"=w1157) -> ("error out"=w1161:errorcluster)  [unwired: 13 in]
                      n314 = local write "STATUS"(w1168) -> ()
                      n315 = call "Delay T4.vi"("milliseconds to wait"=u32 10, "error in (no error)"=w1161) -> ("error out"=w1165:errorcluster)  [unwired: 9 in]
                      n316 = call "WS1050 AD7747 READ.vi"("error in"=w1165, "Log (T)"=FALSE, "DUT Mask Mode (All)"=WSVCAP_SHL_I2C_DUT_Mask_Mode_Enum."C2") -> ("error out"=w1163:errorcluster, "AD7747 Values"=w1164:string[][])  [unwired: 7 in]
                      n317 = for {
                        tunnel: w1164 -> [w1177] mode=indexing
                        tunnel: w1163 -> [w1178]
                        tunnel: [w1178] -> w1159
                        tunnel: [w1175] -> w1167 mode=indexing
                        n318 = Index Array(array=w1177, index=3) -> (element=w1175:string)
                      }
                      n319 = Unbundle By Name(w1159) -> ("status"=w1173:bool)
                      n320 = Or(x=w1173, y=w1172) -> (x .or. y?=w1171:bool)
                    }
                  }
                  frame 1 {
                    n321 = for {
                      N: w1186 -> [_]
                      tunnel: w1183 -> [w1204]
                      tunnel: w1182 -> [w1202]
                      tunnel: [w1201] -> w1181
                      tunnel: [w1197] -> w1184 mode=indexing
                      tunnel: w1185 -> [w1199]
                      tunnel: w1179 -> [w1187]
                      tunnel: [w1189] -> w1180
                      i -> [w1196]
                      stop <- w1201 stop-if-true
                      n322 = Index Array(array=w1204, index=w1196) -> (element=w1200:string)
                      n323 = Index Array(array=w1199, index=w1196) -> (element=w1198:string)
                      n324 = call "WSVCAP SHL Host TL RFFE Write - Multiple DUTs - Common Data.vi"("Data Out"=w1200, "error in"=w1187) -> ("error out"=w1191:errorcluster)  [unwired: 13 in]
                      n325 = local write "STATUS"(w1198) -> ()
                      n326 = call "Delay T4.vi"("milliseconds to wait"=u32 10, "error in (no error)"=w1191) -> ("error out"=w1195:errorcluster)  [unwired: 9 in]
                      n327 = call "WS1050 AD7747 READ.vi"("error in"=w1195, "Log (T)"=FALSE, "DUT Mask Mode (All)"=WSVCAP_SHL_I2C_DUT_Mask_Mode_Enum."C1") -> ("error out"=w1193:errorcluster, "AD7747 Values"=w1194:string[][])  [unwired: 7 in]
                      n328 = for {
                        tunnel: w1194 -> [w1207] mode=indexing
                        tunnel: w1193 -> [w1208]
                        tunnel: [w1208] -> w1189
                        tunnel: [w1205] -> w1197 mode=indexing
                        n329 = Index Array(array=w1207, index=1) -> (element=w1205:string)
                      }
                      n330 = Unbundle By Name(w1189) -> ("status"=w1203:bool)
                      n331 = Or(x=w1203, y=w1202) -> (x .or. y?=w1201:bool)
                    }
                  }
                }
                n332 = Transpose 2D Array(2D array=w1137) -> (transposed array=w1129:string[][])
                "40V_2" <- w1129
              }
              frame #3 {
                n333 = case shown="True" w1211 {
                  tunnel: w1224 -> [_ w1247]
                  tunnel: w1223 -> [_ w1246]
                  tunnel: w1222 -> [w1239 w1241]
                  tunnel: [w1239 w1245] -> w1221
                  tunnel: [string[][] [] w1244] -> w1217
                  tunnel: w1216 -> [w1237 w1243]
                  tunnel: [w1237 w1242] -> w1215
                  tunnel: w1210 -> [_ w1240]
                  frame False {
                  }
                  frame True {
                    n334 = Array Size(array=w1247) -> (size(s)=w1248:i32)
                    n335 = case shown="2" w1240 {
                      tunnel: w1248 -> [w1257 w1288]
                      tunnel: w1247 -> [w1256 w1287]
                      tunnel: w1246 -> [w1255 w1286]
                      tunnel: [w1254 w1285] -> w1245
                      tunnel: [w1252 w1283] -> w1244
                      tunnel: w1243 -> [w1251 w1282]
                      tunnel: [w1250 w1281] -> w1242
                      tunnel: w1241 -> [w1249 w1280]
                      frame 0, 1, Default {
                        n336 = for {
                          N: w1257 -> [_]
                          tunnel: w1255 -> [w1275]
                          tunnel: w1249 -> [w1273]
                          tunnel: [w1272] -> w1254
                          tunnel: [w1268] -> w1253 mode=indexing
                          tunnel: w1256 -> [w1270]
                          tunnel: w1251 -> [w1258]
                          tunnel: [w1260] -> w1250
                          i -> [w1267]
                          stop <- w1272 stop-if-true
                          n337 = Index Array(array=w1275, index=w1267) -> (element=w1271:string)
                          n338 = Index Array(array=w1270, index=w1267) -> (element=w1269:string)
                          n339 = local write "STATUS"(w1269) -> ()
                          n340 = call "WSVCAP SHL Host TL RFFE Write - Multiple DUTs - Common Data.vi"("Data Out"=w1271, "error in"=w1258) -> ("error out"=w1262:errorcluster)  [unwired: 13 in]
                          n341 = call "Delay T4.vi"("milliseconds to wait"=u32 10, "error in (no error)"=w1262) -> ("error out"=w1266:errorcluster)  [unwired: 9 in]
                          n342 = call "WS1050 AD7747 READ.vi"("error in"=w1266, "Log (T)"=FALSE, "DUT Mask Mode (All)"=WSVCAP_SHL_I2C_DUT_Mask_Mode_Enum."C3") -> ("error out"=w1264:errorcluster, "AD7747 Values"=w1265:string[][])  [unwired: 7 in]
                          n343 = for {
                            tunnel: w1265 -> [w1278] mode=indexing
                            tunnel: w1264 -> [w1279]
                            tunnel: [w1279] -> w1260
                            tunnel: [w1276] -> w1268 mode=indexing
                            n344 = Index Array(array=w1278, index=5) -> (element=w1276:string)
                          }
                          n345 = Unbundle By Name(w1260) -> ("status"=w1274:bool)
                          n346 = Or(x=w1274, y=w1273) -> (x .or. y?=w1272:bool)
                        }
                        n347 = Transpose 2D Array(2D array=w1253) -> (transposed array=w1252:string[][])
                      }
                      frame 2 {
                        n348 = for {
                          N: w1288 -> [_]
                          tunnel: w1286 -> [w1306]
                          tunnel: w1280 -> [w1304]
                          tunnel: [w1303] -> w1285
                          tunnel: [w1299] -> w1284 mode=indexing
                          tunnel: w1287 -> [w1301]
                          tunnel: w1282 -> [w1289]
                          tunnel: [w1291] -> w1281
                          i -> [w1298]
                          stop <- w1303 stop-if-true
                          n349 = Index Array(array=w1306, index=w1298) -> (element=w1302:string)
                          n350 = Index Array(array=w1301, index=w1298) -> (element=w1300:string)
                          n351 = local write "STATUS"(w1300) -> ()
                          n352 = call "WSVCAP SHL Host TL RFFE Write - Multiple DUTs - Common Data.vi"("Data Out"=w1302, "error in"=w1289) -> ("error out"=w1293:errorcluster)  [unwired: 13 in]
                          n353 = call "Delay T4.vi"("milliseconds to wait"=u32 10, "error in (no error)"=w1293) -> ("error out"=w1297:errorcluster)  [unwired: 9 in]
                          n354 = call "WS1050 AD7747 READ.vi"("error in"=w1297, "Log (T)"=FALSE, "DUT Mask Mode (All)"=WSVCAP_SHL_I2C_DUT_Mask_Mode_Enum."C1") -> ("error out"=w1295:errorcluster, "AD7747 Values"=w1296:string[][])  [unwired: 7 in]
                          n355 = for {
                            tunnel: w1296 -> [w1309] mode=indexing
                            tunnel: w1295 -> [w1310]
                            tunnel: [w1310] -> w1291
                            tunnel: [w1307] -> w1299 mode=indexing
                            n356 = Index Array(array=w1309, index=1) -> (element=w1307:string)
                          }
                          n357 = Unbundle By Name(w1291) -> ("status"=w1305:bool)
                          n358 = Or(x=w1305, y=w1304) -> (x .or. y?=w1303:bool)
                        }
                        n359 = Transpose 2D Array(2D array=w1284) -> (transposed array=w1283:string[][])
                      }
                    }
                  }
                }
                "40V_3" <- w1217
                n360 = case shown="False" w1211 {
                  tunnel: ["DeltaC Target(pF)_51" "DeltaC Target(pF)_50"] -> w1220
                  frame False {
                  }
                  frame True {
                  }
                }
              }
              frame #4 {
                # "VPI Testing @ 35V"
                n361 = call "WS1050 Delta C Calculation.vi"("WS1050/51"=w1314, "error in (no error)"=w1349, "DCap Target(pF)"=w1348, "Input"=w1351) -> ("error out"=w1346:errorcluster, "Total Bank Delta C(pF)"=w1339:string[], "% Bank DeltaC"=w1343:string[])  [unwired: 3 in, 2 out]
                n362 = call "WS1050 Delta C Calculation.vi"("WS1050/51"=w1313, "error in (no error)"=w1349, "DCap Target(pF)"=w1348, "Input"=w1350) -> ("error out"=w1347:errorcluster, "Total Bank Delta C(pF)"=w1338:string[], "% Bank DeltaC"=w1341:string[])  [unwired: 3 in, 2 out]
                n363 = call "WS1050 Delta C Calculation.vi"("WS1050/51"=w1312, "error in (no error)"=w1349, "DCap Target(pF)"=w1348, "Input"=w1342) -> ("error out"=w1345:errorcluster, "Total Bank Delta C(pF)"=w1337:string[], "% Bank DeltaC"=w1340:string[])  [unwired: 3 in, 2 out]
                n364 = Merge Errors(w1346, w1347, w1345) -> (w1344:errorcluster)
                n365 = case shown="1, Default" w1352 {
                  tunnel: w1344 -> [w1380 w1388]
                  tunnel: [w1380 w1388] -> w1316
                  tunnel: w1343 -> [w1376 w1384]
                  tunnel: w1341 -> [w1375 w1383]
                  tunnel: w1340 -> [w1374 w1382]
                  tunnel: w1339 -> [w1379 w1387]
                  tunnel: [w1379 w1387] -> w1336
                  tunnel: w1338 -> [w1378 w1386]
                  tunnel: [w1378 w1386] -> w1335
                  tunnel: w1337 -> [w1377 w1385]
                  tunnel: [w1377 w1385] -> w1334
                  frame 0 {
                    n366 = Build Array(w1376, w1375, w1374) -> (→"% Delta C_T0":string[][])
                  }
                  frame 1, Default {
                    n367 = Build Array(w1384, w1383, w1382) -> (→"% Delta C":string[][])
                  }
                }
                "Total Delta 1(pF)" <- w1336
                "Total Delta 2(pF)" <- w1335
                "Total Delta 3(pF)" <- w1334
                n368 = call "Multi Dut Cmd VPI Setting.vi"("error in (no error)"=w1316, "Cmin/Act"=w1311, "WS1050/51"=w1314) -> ("error out"=w1315:errorcluster, "Cmd VPI C3"=w1317:string[], "VPI_C3"=w1321:string[], "Name Header VPI"=w1320:string[], "Cmd VPI C2"=w1318:string[], "VPI_C2"=w1322:string[], "Cmd VPI C1"=w1319:string[], "VPI_C1"=w1323:string[])  [unwired: 1 in]
                n369 = case shown="False" w1326 {
                  tunnel: w1366 -> [w1394 w1424]
                  tunnel: [w1393 w1405] -> w1330
                  tunnel: [w1391 w1426] -> w1365
                  tunnel: [w1391 w1412] -> w1364
                  tunnel: [w1394 w1410] -> w1362
                  tunnel: w1359 -> [w1396 w1425]
                  tunnel: [w1396 w1425] -> w1358
                  tunnel: w1319 -> [_ w1423]
                  tunnel: w1318 -> [_ w1417]
                  tunnel: w1317 -> [_ w1413]
                  tunnel: [w1391 w1422] -> w1355
                  tunnel: w1323 -> [w1389 w1420]
                  tunnel: w1322 -> [_ w1418]
                  tunnel: w1321 -> [_ w1414]
                  tunnel: ["NA" ("string") w1409] -> w1332
                  tunnel: w1315 -> [w1393 w1401]
                  tunnel: w1314 -> [_ w1400]
                  frame False {
                    n370 = Array Size(array=w1389) -> (size(s)=w1390:i32)
                    n371 = for {
                      N: w1390 -> [_]
                      tunnel: [w1397] -> w1392 mode=indexing
                      n372 = for {
                        N: 16 -> [_]
                        tunnel: ["na"] -> w1397 mode=indexing
                      }
                    }
                    n373 = Transpose 2D Array(2D array=w1392) -> (transposed array=w1391:string[][])
                    n374 = local write "VPI C1"(w1391) -> ()
                    n375 = local write "VPI C2"(w1391) -> ()
                    n376 = local write "VPI C3"(w1391) -> ()
                  }
                  frame True {
                    # "Set CP to 35V"
                    n377 = flat-sequence {
                      tunnel: [w1486] -> w1406
                      tunnel: w1401 -> [w1484]
                      tunnel: [w1491] -> w1409
                      tunnel: w1406 -> [w1490]
                      tunnel: [w1489] -> w1404
                      frame #0 {
                        n378 = call "WSVCAP SHL Host TL RFFE Write - Multiple DUTs - Common Data.vi"("Data Out"="074820", "error in"=w1484) -> ("error out"=w1487:errorcluster)  [unwired: 13 in]
                        n379 = call "Delay T4.vi"("milliseconds to wait"=u32 10, "error in (no error)"=w1487) -> ("error out"=w1486:errorcluster)  [unwired: 9 in]
                      }
                      frame #1 {
                        n380 = case shown="4" "CP VPI" {
                          selector: "CP VPI" -> [w1499 w1504 w1509 w1514 w1518]
                          tunnel: string[] ["07476F", "074776", "074765", "074769", "07477B"] -> [w1500 w1505 w1510 w1515 w1520]
                          tunnel: [w1498 w1503 w1508 w1513 w1519] -> w1494
                          tunnel: [w1496 w1501 w1506 w1511 w1516] -> w1493
                          tunnel: ["35" ("string") "27.5" ("string") "30.5" ("string") "44.0" ("string") "40.25" ("string")] -> w1491
                          tunnel: w1490 -> [w1496 w1501 w1506 w1511 w1516]
                          frame 0, Default {
                            n381 = Index Array(array=w1500, index=w1499) -> (element=w1498:string)
                          }
                          frame 2 {
                            n382 = Index Array(array=w1505, index=w1504) -> (element=w1503:string)
                          }
                          frame 3 {
                            n383 = Index Array(array=w1510, index=w1509) -> (element=w1508:string)
                          }
                          frame 4 {
                            n384 = Index Array(array=w1515, index=w1514) -> (element=w1513:string)
                          }
                          frame 1 {
                            n385 = Index Array(array=w1520, index=w1518) -> (element=w1519:string)
                          }
                        }
                        n386 = call "WSVCAP SHL Host TL RFFE Write - Multiple DUTs - Common Data.vi"("Data Out"=w1494, "error in"=w1493) -> ("error out"=w1489:errorcluster)  [unwired: 13 in]
                      }
                    }
                    n387 = Array Size(array=w1420) -> (size(s)=w1427:i32)
                    n388 = call "Delay T4.vi"("milliseconds to wait"=u32 50, "error in (no error)"=w1404) -> ("error out"=w1403:errorcluster)  [unwired: 9 in]
                    n389 = for {
                      N: w1427 -> [_]
                      tunnel: w1423 -> [w1538]
                      tunnel: w1424 -> [w1536]
                      tunnel: [w1535] -> w1416
                      tunnel: [w1533] -> w1421 mode=indexing
                      tunnel: w1420 -> [w1532]
                      tunnel: w1403 -> [w1521]
                      tunnel: [w1523] -> w1408
                      i -> [w1531]
                      stop <- w1535 stop-if-true
                      n390 = Index Array(array=w1538, index=w1531) -> (element=w1534:string)
                      n391 = Index Array(array=w1532, index=w1531) -> (element=w1530:string)
                      n392 = call "WSVCAP SHL Host TL RFFE Write - Multiple DUTs - Common Data.vi"("Data Out"=w1534, "error in"=w1521) -> ("error out"=w1529:errorcluster)  [unwired: 13 in]
                      n393 = local write "STATUS"(w1530) -> ()
                      n394 = call "Delay T4.vi"("milliseconds to wait"=u32 10, "error in (no error)"=w1529) -> ("error out"=w1525:errorcluster)  [unwired: 9 in]
                      n395 = call "WS1050 AD7747 READ.vi"("error in"=w1525, "Log (T)"=FALSE, "DUT Mask Mode (All)"=WSVCAP_SHL_I2C_DUT_Mask_Mode_Enum."C1") -> ("error out"=w1527:errorcluster, "AD7747 Values"=w1526:string[][])  [unwired: 7 in]
                      n396 = for {
                        tunnel: [w1541] -> w1533 mode=indexing
                        tunnel: w1527 -> [w1540]
                        tunnel: [w1540] -> w1523
                        tunnel: w1526 -> [w1539] mode=indexing
                        n397 = Index Array(array=w1539, index=1) -> (element=w1541:string)
                      }
                      n398 = Unbundle By Name(w1523) -> ("status"=w1537:bool)
                      n399 = Or(x=w1537, y=w1536) -> (x .or. y?=w1535:bool)
                    }
                    n400 = Transpose 2D Array(2D array=w1421) -> (transposed array=w1426:string[][])
                    "VPI C1" <- w1426
                    n401 = Array Size(array=w1418) -> (size(s)=w1419:i32)
                    n402 = for {
                      N: w1419 -> [_]
                      tunnel: w1417 -> [w1479]
                      tunnel: w1416 -> [w1477]
                      tunnel: [w1476] -> w1411
                      tunnel: [w1474] -> w1415 mode=indexing
                      tunnel: w1418 -> [w1473]
                      tunnel: w1408 -> [w1462]
                      tunnel: [w1464] -> w1407
                      i -> [w1472]
                      stop <- w1476 stop-if-true
                      n403 = Index Array(array=w1479, index=w1472) -> (element=w1475:string)
                      n404 = Index Array(array=w1473, index=w1472) -> (element=w1471:string)
                      n405 = call "WSVCAP SHL Host TL RFFE Write - Multiple DUTs - Common Data.vi"("Data Out"=w1475, "error in"=w1462) -> ("error out"=w1470:errorcluster)  [unwired: 13 in]
                      n406 = local write "STATUS"(w1471) -> ()
                      n407 = call "Delay T4.vi"("milliseconds to wait"=u32 10, "error in (no error)"=w1470) -> ("error out"=w1466:errorcluster)  [unwired: 9 in]
                      n408 = call "WS1050 AD7747 READ.vi"("error in"=w1466, "Log (T)"=FALSE, "DUT Mask Mode (All)"=WSVCAP_SHL_I2C_DUT_Mask_Mode_Enum."C2") -> ("error out"=w1468:errorcluster, "AD7747 Values"=w1467:string[][])  [unwired: 7 in]
                      n409 = for {
                        tunnel: [w1482] -> w1474 mode=indexing
                        tunnel: w1468 -> [w1481]
                        tunnel: [w1481] -> w1464
                        tunnel: w1467 -> [w1480] mode=indexing
                        n410 = Index Array(array=w1480, index=3) -> (element=w1482:string)
                      }
                      n411 = Unbundle By Name(w1464) -> ("status"=w1478:bool)
                      n412 = Or(x=w1478, y=w1477) -> (x .or. y?=w1476:bool)
                    }
                    n413 = Transpose 2D Array(2D array=w1415) -> (transposed array=w1422:string[][])
                    "VPI C2" <- w1422
                    n414 = case shown="True" w1400 {
                      tunnel: w1414 -> [_ w1438]
                      tunnel: w1413 -> [_ w1437]
                      tunnel: [string[][] [] w1435] -> w1412
                      tunnel: w1411 -> [w1430 w1434]
                      tunnel: [w1430 w1433] -> w1410
                      tunnel: w1407 -> [w1429 w1432]
                      tunnel: [w1429 w1431] -> w1405
                      frame False {
                      }
                      frame True {
                        n415 = Array Size(array=w1438) -> (size(s)=w1439:i32)
                        n416 = for {
                          N: w1439 -> [_]
                          tunnel: w1437 -> [w1457]
                          tunnel: w1434 -> [w1455]
                          tunnel: [w1454] -> w1433
                          tunnel: [w1452] -> w1436 mode=indexing
                          tunnel: w1438 -> [w1451]
                          tunnel: w1432 -> [w1440]
                          tunnel: [w1442] -> w1431
                          i -> [w1450]
                          stop <- w1454 stop-if-true
                          n417 = Index Array(array=w1457, index=w1450) -> (element=w1453:string)
                          n418 = Index Array(array=w1451, index=w1450) -> (element=w1449:string)
                          n419 = call "WSVCAP SHL Host TL RFFE Write - Multiple DUTs - Common Data.vi"("Data Out"=w1453, "error in"=w1440) -> ("error out"=w1448:errorcluster)  [unwired: 13 in]
                          n420 = local write "STATUS"(w1449) -> ()
                          n421 = call "Delay T4.vi"("milliseconds to wait"=u32 10, "error in (no error)"=w1448) -> ("error out"=w1444:errorcluster)  [unwired: 9 in]
                          n422 = call "WS1050 AD7747 READ.vi"("error in"=w1444, "Log (T)"=FALSE, "DUT Mask Mode (All)"=WSVCAP_SHL_I2C_DUT_Mask_Mode_Enum."C3") -> ("error out"=w1446:errorcluster, "AD7747 Values"=w1445:string[][])  [unwired: 7 in]
                          n423 = for {
                            tunnel: [w1460] -> w1452 mode=indexing
                            tunnel: w1446 -> [w1459]
                            tunnel: [w1459] -> w1442
                            tunnel: w1445 -> [w1458] mode=indexing
                            n424 = Index Array(array=w1458, index=5) -> (element=w1460:string)
                          }
                          n425 = Unbundle By Name(w1442) -> ("status"=w1456:bool)
                          n426 = Or(x=w1456, y=w1455) -> (x .or. y?=w1454:bool)
                        }
                        n427 = Transpose 2D Array(2D array=w1436) -> (transposed array=w1435:string[][])
                      }
                    }
                    "VPI C3" <- w1412
                  }
                }
                n428 = Insert Into Array(array=w1354, new element=w1320) -> (w1353:string[])  [unwired: 1 in]
                n429 = case shown="False" w1331 {
                  tunnel: w1330 -> [w1367 w1371]
                  tunnel: [w1368 w1370] -> w1329
                  frame False {
                    n430 = call "WSVCAP SHL Host TL RFFE Write - Multiple DUTs - Common Data.vi"("Data Out"="074820", "error in"=w1367) -> ("error out"=w1368:errorcluster)  [unwired: 13 in]
                  }
                  frame True {
                    n431 = call "WSVCAP SHL Host TL RFFE Write - Multiple DUTs - Common Data.vi"("Data Out"="074800", "error in"=w1371) -> ("error out"=w1370:errorcluster)  [unwired: 13 in]
                  }
                }
                n432 = call "Delay T4.vi"("milliseconds to wait"=u32 50, "error in (no error)"=w1329) -> ("error out"=w1328:errorcluster)  [unwired: 9 in]
              }
              frame #5 {
                # "VSA Testing"
                n433 = case shown="False" w1544 {
                  tunnel: w1583 -> [w1598 w1607]
                  tunnel: [w1598 w1606] -> w1557
                  tunnel: [w1597 w1613] -> w1573
                  tunnel: w1574 -> [w1597 w1612]
                  tunnel: [w1594 w1610] -> w1562
                  tunnel: [w1594 w1609] -> w1559
                  tunnel: [w1594 w1608] -> w1556
                  tunnel: [w1595 w1611] -> w1563
                  frame False {
                    n434 = for {
                      tunnel: dbl[] [0.0, 0.0, 0.0] -> [w1602] mode=indexing
                      tunnel: [w1600] -> w1595 mode=indexing
                      tunnel: [w1599] -> w1594 mode=indexing
                      n435 = Number To Fractional String(number=w1602) -> (F-format string=w1601:string)  [unwired: 3 in]
                      n436 = for {
                        N: 16 -> [_]
                        tunnel: w1601 -> [w1605]
                        tunnel: [w1605] -> w1600 mode=indexing
                        tunnel: ["na"] -> w1599 mode=indexing
                      }
                    }
                  }
                  frame True {
                    n437 = for {
                      tunnel: "VSA Voltage(V)" -> [w1637] mode=indexing
                      tunnel: [w1641] -> w1613
                      tunnel: w1612 -> [w1639]
                      tunnel: [w1638] -> w1610 mode=indexing
                      tunnel: [w1625] -> w1609 mode=indexing
                      tunnel: [w1634] -> w1611 mode=indexing
                      tunnel: [w1619] -> w1608 mode=indexing
                      tunnel: w1607 -> [w1618]
                      tunnel: [w1617] -> w1606
                      w1616 = FALSE ("Log (T)")
                      w1633 = u16 0 items=["Voltage", "Current"] ("Source Mode  (0: Voltage)")
                      n438 = call "Configure Output.vi"("Source Mode  (0: Voltage)"=w1633, "error in (no error)"=w1618, "Compliance  Level (0.1)"=0.1, "Output Level (0)"=w1637, "VISA resource name"=w1639) -> ("error out"=w1645:errorcluster, "VISA resource name out"=w1643:refnum<visa-resource-name>)  [unwired: 5 in]
                      n439 = Number To Fractional String(number=w1637) -> (F-format string=w1636:string)  [unwired: 3 in]
                      n440 = call "Enable Output.vi"("error in (no error)"=w1645, "Enable Output (T: Enable)"=TRUE, "VISA resource name"=w1643) -> ("error out"=w1646:errorcluster, "VISA resource name out"=w1641:refnum<visa-resource-name>)  [unwired: 7 in]
                      n441 = call "Delay T4.vi"("milliseconds to wait"=u32 10, "error in (no error)"=w1646) -> ("error out"=w1632:errorcluster)  [unwired: 9 in]
                      n442 = call "WS1050 AD7747 READ.vi"("error in"=w1632, "Log (T)"=w1616, "DUT Mask Mode (All)"=WSVCAP_SHL_I2C_DUT_Mask_Mode_Enum."C1") -> ("error out"=w1629:errorcluster, "AD7747 Values"=w1631:string[][])  [unwired: 7 in]
                      n443 = for {
                        tunnel: w1631 -> [w1657] mode=indexing
                        tunnel: [w1658] -> w1638 mode=indexing
                        tunnel: w1629 -> [w1656]
                        tunnel: [w1656] -> w1628
                        n444 = Index Array(array=w1657, index=1) -> (element=w1658:string)
                      }
                      n445 = for {
                        N: 16 -> [_]
                        tunnel: w1636 -> [w1655]
                        tunnel: [w1655] -> w1634 mode=indexing
                      }
                      n446 = call "WS1050 AD7747 READ.vi"("error in"=w1628, "Log (T)"=w1616, "DUT Mask Mode (All)"=WSVCAP_SHL_I2C_DUT_Mask_Mode_Enum."C2") -> ("error out"=w1626:errorcluster, "AD7747 Values"=w1624:string[][])  [unwired: 7 in]
                      n447 = for {
                        tunnel: w1624 -> [w1652] mode=indexing
                        tunnel: [w1653] -> w1625 mode=indexing
                        tunnel: w1626 -> [w1651]
                        tunnel: [w1651] -> w1623
                        n448 = Index Array(array=w1652, index=3) -> (element=w1653:string)
                      }
                      n449 = call "WS1050 AD7747 READ.vi"("error in"=w1623, "Log (T)"=w1616, "DUT Mask Mode (All)"=WSVCAP_SHL_I2C_DUT_Mask_Mode_Enum."C3") -> ("error out"=w1621:errorcluster, "AD7747 Values"=w1620:string[][])  [unwired: 7 in]
                      n450 = for {
                        tunnel: w1620 -> [w1648] mode=indexing
                        tunnel: [w1649] -> w1619 mode=indexing
                        tunnel: w1621 -> [w1647]
                        tunnel: [w1647] -> w1617
                        n451 = Index Array(array=w1648, index=5) -> (element=w1649:string)
                      }
                    }
                    n452 = local write "STATUS"("VSA Testing...." ("STATUS")) -> ()
                  }
                }
                n453 = Transpose 2D Array(2D array=w1563) -> (transposed array=w1561:string[][])
                n454 = Transpose 2D Array(2D array=w1562) -> (transposed array=w1560:string[][])
                n455 = Transpose 2D Array(2D array=w1559) -> (transposed array=w1558:string[][])
                n456 = Transpose 2D Array(2D array=w1556) -> (transposed array=w1555:string[][])
                n457 = call "WS1050_VSA_Convert_Data Updated.vi"("VSA_C3"=w1555, "WS1050/51"=w1543, "error in (no error)"=w1557, "VSA_C2"=w1558, "VSA_C1"=w1560, "Voltage"=w1561) -> ("error out"=w1554:errorcluster, "VSA_V3"=w1551:string[][], "VSA_V2"=w1552:string[][], "VSA_V1"=w1553:string[][])  [unwired: 2 in]
                "VSA_V1" <- w1553
                "VSA_V2" <- w1552
                "VSA_V3" <- w1551
                n458 = case shown="True" w1544 {
                  tunnel: w1573 -> [w1587 w1593]
                  tunnel: [w1587 w1592] -> w1572
                  tunnel: w1554 -> [w1586 w1591]
                  tunnel: [w1586 w1588] -> w1571
                  frame False {
                  }
                  frame True {
                    w1589 = u16 0 items=["Voltage", "Current"] ("Source Mode  (0: Voltage)")
                    n459 = call "Configure Output.vi"("Source Mode  (0: Voltage)"=w1589, "error in (no error)"=w1591, "Output Level (0)"=0.0, "VISA resource name"=w1593) -> ("error out"=w1588:errorcluster, "VISA resource name out"=w1592:refnum<visa-resource-name>)  [unwired: 6 in]
                  }
                }
                n460 = call "Delay T4.vi"("milliseconds to wait"=u32 50, "error in (no error)"=w1571) -> ("error out"=w1570:errorcluster)  [unwired: 9 in]
              }
              frame #6 {
                # "Handshake Check and EFuse Readback"
                n461 = Or(x=w1669, y=w1679) -> (x .or. y?=w1678:bool)
                n462 = Add(x=w1691, y=w1690) -> (x+y=w1677:u64)
                n463 = case shown="True" w1678 {
                  tunnel: w1704 -> [w1717 _]
                  tunnel: w1703 -> [w1716 w1721]
                  tunnel: [w1715 w1721] -> w1702
                  tunnel: w1701 -> [w1714 _]
                  tunnel: w1700 -> [w1713 _]
                  tunnel: w1699 -> [w1712 _]
                  tunnel: [w1708 w1720] -> w1698
                  tunnel: [w1707 w1720] -> w1693
                  tunnel: w1677 -> [w1706 _]
                  tunnel: w1684 -> [w1705 _]
                  frame False {
                    n464 = call "WS1050_16DUT_Handshake Check R1_Record All Regs Ver1.0.vi"("file path (use dialog)"=w1717, "Reg1_Bit Cntrl"="Reg1_Bit Cntrl", "File Name"=w1705, "SN"=w1712, "Loop"=w1706, "error"=w1716, "Lot #"=w1714, "Wafer #"=w1713) -> ("Pass/Fail"=→"EFuse Readback Status":bool[], "EFuse Read back"=w1707:string[], "Status"=w1708:string[], "error out"=w1715:errorcluster)  [unwired: 6 in, 2 out]
                    n465 = case shown="1, Default" w1706 {
                      tunnel: w1707 -> [w1718 w1719]
                      frame 0 {
                        "EFuse RB T0" <- w1718
                      }
                      frame 1, Default {
                        "Current EFuse Read back" <- w1719
                      }
                    }
                    n466 = local write "STATUS"("Hand Shake & EFuse Readback...." ("STATUS")) -> ()
                  }
                  frame True {
                    w1720 = string[] ["NA", "NA", "NA", "NA", "NA", "NA", "NA", "NA", "NA", "NA", "NA", "NA", "NA", "NA", "NA", "NA"] ("EFuse Read back")
                  }
                }
                n467 = Add(x=w1677, y=w1674) -> (x+y=w1675:u64)
                "TTime Completed" <- w1675
                n468 = Number To Engineering String(4:w1675) -> (0:w1689:string)  [unwired: 3 in]
                n469 = Build Array(w1688, w1686, w1685) -> (w1687:string[])
              }
              frame #7 {
                # "Save Data"
                n470 = Increment(x=w1732) -> (x+1=w1731:i32)
                n471 = local write "STATUS"("Saving Data...." ("STATUS")) -> ()
                n472 = Multiply(x=w1731, y=16) -> (x*y=w1726:i32)
                n473 = Path To String(path=w1736) -> (string=w1735:string)
                n474 = Bundle("Test Program"=w1769, "Comment"=w1768, "Data Out"=w1744, "Data Out"=w1742, "Data Out"=w1741, w1740, "Data Out"=w1739, "Data Out"=w1738, "string"=w1737, "Freq(Hz)"=w1724, "Brd #"=w1723) -> (w1743:T8)  [unwired: 1 in]
                n475 = case shown="True" "Debug" {
                  tunnel: w1726 -> [w1776 w1779]
                  tunnel: [w1776 w1777] -> w1725
                  frame False {
                  }
                  frame True {
                    n476 = Multiply(x=w1779, y="No of Rows\nFrom Spread Sheet") -> (x*y=w1777:i32)
                  }
                }
                n477 = call "WS1050_16 DUT SData ver1.3"("TMN DC\\CAP Data Log File Path"=w1736, "Lot#"=w1771, "Total Delta C1(pF)"=w1747, "VSA_V1"=w1756, "Wafer#"=w1767, "File Name"=w1729, "Total Delta C2(pF)"=w1746, "error in"=w1774, "TP/Comment"=w1743, "EFuse"=w1761, "Data Output C3"=w1749, "Temperature"=w1753, "VSA_V2"=w1757, "VPI C3"=w1751, "Data Output C1"=w1764, "VPI C2"=w1750, "SN"=w1772, "R/W Status"=w1770, "Cap Header"=w1752, "HD/Cycles Completed"=w1760, "Data Output C2"=w1748, "VSA_V3"=w1755, "Current"=w1763, "VPI C1"=w1762, "Total Delta C3(pF)"=w1745) -> ("error out"=w1773:errorcluster)  [unwired: 2 in]
                n478 = Concatenate Strings(w1735, "\\" ("string"), w1729, "_Multi Socket Data.csv" ("string")) -> (w1734:string)
              }
              frame #8 {
                n479 = case shown="True" "Plot Delta Cmin" {
                  tunnel: w1785 -> [w1800 w1816]
                  tunnel: [w1800 w1812] -> w1784
                  tunnel: w1783 -> [_ w1808]
                  tunnel: w1781 -> [_ w1806]
                  tunnel: w1780 -> [_ w1801]
                  frame False {
                  }
                  frame True {
                    n480 = String To Path(string=w1808) -> (path=w1807:path)
                    n481 = call "Delay T4.vi"("milliseconds to wait"=u32 50, "error in (no error)"=w1816) -> ("error out"=w1815:errorcluster)  [unwired: 9 in]
                    n482 = call "16DUT Plot Subvi Ver1.0.vi"("Plot"="Plot", "No of Rows"=w1806, "error in (no error)"=w1815, "WS1050/51"=w1801, "Bank"=enum16{"C1", "C2", "C3"}."C1", "file path (dialog if empty)"=w1807) -> ("error out"=w1810:errorcluster, "Delta C_Min Plot"=→"Min Plot_1":dbl[][])  [unwired: 4 in]
                    n483 = call "16DUT Plot Subvi Ver1.0.vi"("Plot"="Plot", "No of Rows"=w1806, "error in (no error)"=w1810, "WS1050/51"=w1801, "Bank"=enum16{"C1", "C2", "C3"}."C2", "file path (dialog if empty)"=w1807) -> ("error out"=w1811:errorcluster, "Delta C_Min Plot"=→"Min Plot_2":dbl[][])  [unwired: 4 in]
                    n484 = call "16DUT Plot Subvi Ver1.0.vi"("Plot"="Plot", "No of Rows"=w1806, "error in (no error)"=w1811, "WS1050/51"=w1801, "Bank"=enum16{"C1", "C2", "C3"}."C3", "file path (dialog if empty)"=w1807) -> ("error out"=w1812:errorcluster, "Delta C_Min Plot"=→"Min Plot_3":dbl[][])  [unwired: 4 in]
                  }
                }
                n485 = Get Date/Time In Seconds() -> (seconds since 1Jan1904=w1793:timestamp)
                n486 = Get Date/Time String(seconds (now)=w1793, want seconds? (F)=TRUE) -> (date string=→"date string":string, time string=→"Previous Time":string)  [unwired: 1 in]
                n487 = Greater Or Equal?(x=w1789, y="TTF Completed") -> (x >= y?=w1788:bool)
                n488 = Greater Or Equal?(x=w1790, y="Set HD/Cycle \nto Complete") -> (x >= y?=w1797:bool)
                "No of HD/Cycle\nCompleted" <- w1790
              }
            }
            n489 = Increment(x=w535) -> (x+1=→"Loop \ncompleted":i32)
            n490 = call "Delay T4.vi"("milliseconds to wait"=u32 50, "error in (no error)"=w422) -> ("error out"=w423:errorcluster)  [unwired: 9 in]
            n491 = Compound Arithmetic op=OR(w607, w505, w531) -> (w544:bool)
          }
          "Total Time" <- w363
          n492 = Increment(x=w361) -> (x+1=→"Running Loops":i32)
          n493 = local write "No of HD/Cycle\nCompleted"(u64 0 ("No of HD/Cycle\nCompleted")) -> ()
          n494 = Unbundle By Name(w354) -> ("status"=w367:bool)
          n495 = Compound Arithmetic op=OR(w367, w342, w359) -> (w350:bool)
        }
        n496 = for {
          tunnel: w277 -> [w1827]
          tunnel: w307 -> [w1826]
          tunnel: w308 -> [w1823] mode=indexing
          tunnel: [w1818] -> w275
          tunnel: [w1822] -> w306
          n497 = call "E3631A_Voltage Controller.vi"("VISA resource name"=w1826, "Channel Controller"=w1823, "Voltage 1"=0.0, "Voltage 2"=3.3, "error in (no error)"=w1827, "Voltage 3"=-3.3) -> ("VISA resource name out"=w1822:refnum<visa-resource-name>, "error out"=w1819:errorcluster)  [unwired: 8 in]
          n498 = call "Delay T4.vi"("milliseconds to wait"=u32 100, "error in (no error)"=w1819) -> ("error out"=w1818:errorcluster)  [unwired: 9 in]
        }
        n499 = VISA Write(VISA resource name=w297, write buffer="SOUR:FUNC VOLT;VOLT:MODE FIX;RANG 100;LEV 0.0;:SENS:FUNC \"CURR\";CURR:PROT 60E-3;RANG 100E-3;:OUTP ON", error in (no error)=w277) -> (VISA resource name out=w295:refnum<visa-resource-name>, error out=w276:errorcluster)  [unwired: 1 out]
        n500 = Merge Errors(w275, w276) -> (w296:errorcluster)
      }
      frame True {
      }
    }
    n501 = local write "stop During HD/Cycles"(w53) -> ()
    n502 = Unbundle By Name(w64) -> ("status"=w54:bool)
    n503 = Compound Arithmetic op=OR(w54, w53, w73) -> (w82:bool)
    n504 = Wait Until Next ms Multiple(millisecond multiple=u32 100) -> ()  [unwired: 1 out]
    "STATUS" <- "Idle...." ("STATUS")
  }
  "Ke2000 Out" <- w21
  "PS1 Out" <- w20
  n505 = local write "stop During HD/Cycles"(w6) -> ()
  n506 = local write "stop"(w6) -> ()
  n507 = case shown="True" w18 {
    tunnel: [w1844 w1846] -> w1
    tunnel: w12 -> [w1844 w1845]
    frame False {
    }
    frame True {
      n508 = flat-sequence {
        tunnel: w1845 -> [w1849]
        tunnel: [w1848] -> w1846
        frame #0 {
          n509 = local write "Online"(FALSE ("Online")) -> ()
          n510 = call "WSVCAP SHL Host TL Close.vi"("error in"=w1849) -> ("error out"=w1848:errorcluster)  [unwired: 14 in]
        }
      }
    }
  }
  "error out" <- w1
  n511 = VISA Write(VISA resource name=w13, write buffer="SOUR:FUNC VOLT;VOLT:MODE FIX;RANG 100;LEV 0.0;:SENS:FUNC \"CURR\";CURR:PROT 60E-3;RANG 100E-3;:OUTP OFF", error in (no error)=w12) -> (VISA resource name out=→"VISA resource name out":refnum<visa-resource-name>, error out=→"error out 2":errorcluster)  [unwired: 1 out]
